vi "main.vi"() -> ()   [LabVIEW 2024]
uses:
  DataCluster.ctl
  <vilib>/userDefined/High Color/IMAQdx.ctl
  <vilib>/vision/Image Controls.llb/IMAQ Image.ctl
  <vilib>/Platform/TimedLoop/XDataNode/timing_clust.ctl
  <vilib>/Platform/TimedLoop/XDataNode/nitl_modes.ctl
  <vilib>/Platform/TimedLoop/XDataNode/wakeup.ctl
  4e5cdf46-f112-4ee0-b7be-49a859f3bfc5.vi
  <extravilib>/ChannelInstances/Tag-t'DataCluster.ctl'/Read With Abort.vi
  <extravilib>/ChannelInstances/Tag-t'DataCluster.ctl'/Write With Abort.vi
  <extravilib>/ChannelInstances/Tag-t'DataCluster.ctl'/Instantiate.vi
  <extravilib>/ChannelInstances/Tag-t'DataCluster.ctl'/EndpointRead.vi
  <extravilib>/ChannelInstances/Stream-str/Instantiate.vi
  <extravilib>/ChannelInstances/Tag-c(a[.](dbl),a[.](dbl))/Instantiate.vi
  <vilib>/Platform/browser.llb/Open URL in Default Browser (string).vi
  <extravilib>/ChannelInstances/Tag-t'DataCluster.ctl'/Endpoint.vi
  <vilib>/platform/TimedLoop/XDataNode/XDataNode.xnode
  <vilib>/vision/driver/NI_Vision_Acquisition_Software.lvlib
  <extravilib>/ChannelInstances/Tag-t'DataCluster.ctl'.lvlib
  <vilib>/Platform/TimedLoop/XDataNode/XDNodeRunTimeDep.lvlib
panel:
  out "Cooling label":string
  out "Galium Control":string="Galium Control" caption="Version"
  in  "Freeze":bool
  in  "Melt":bool
  in  "OverlayTemp?":bool
  out "error out 2":errorcluster
  out "T_Left":string="00:30:00" caption="Time Left:"
  out "version":string="version 0.0.0.1" caption="Version"
  in  "Start":bool
  out "Title":string="Ice Nucleation Contoller" caption="Version"
  out "Error Array":errorcluster[](array[cluster])
  out "cDAQ_Time":u32(graph) caption="DAQ - Process Time"
  out "DL_Time":u32(graph) caption="cDAQ - Process Time"
  out "DP_Overhead":i64(graph)=499 caption="Data Acquisition - Overhead"
  in  "DataCluster":T1={"Core"={"Current VI Reference"=refnum, "Close Panel on Exit?"=FALSE, "Exit"=FALSE, "Initialized?"=FALSE}, "Connections"={"cDAQ"={"Task"="", "Connected"=FALSE, "Active"=FALSE, "ID"=""}, "Camera"={"Session"="", "Connected"=FALSE, "Active"=FALSE, "Placeholder"=refnum}, "PSU"={"Port"="", "Connected"=FALSE, "Active"=FALSE}, "Arduino"={"Port"="", "Connected"=FALSE, "Active"=FALSE}}, "Data Acquisition"={"Setup"={"Label"="", "Operator"="", "Notes"="", "TempGrad"=0.0, "TargetTemp"=0.0, "Sample Volume"=1.0}, "Camera"={"Image"=refnum, "Save Image"=refnum, "Image Frequency"=20, "Rectangle"={"Left"=0, "Top"=0, "Right"=0, "Bottom"=0, "Rotation"=0.0}, "Calibration"={"Top Left"={"X"=0.0, "Y"=0.0}, "Top Right"={"X"=0.0, "Y"=0.0}, "Bottom Left"={"X"=0.0, "Y"=0.0}, "Bottom Right"={"X"=0.0, "Y"=0.0}, "Fixpoint"={"X"=0.0, "Y"=0.0}, "Scan Area"=0.0, "Fixpoint Area"=0.0, "Well Pixels"=[], "Valid"=FALSE}, "FocusPos"=0, "Display Mapping"=10, "Camera Mode"=10}, "Thermistor"={"Sample Size"=0, "Calibration"={"B0.100"=[], "R25"=[], "c"=[], "State"=[], "V_S"=0.0, "R_S"=0.0}, "Timing Mode"=14713}, "Partition"={"Data"=[], "Cell Label"="", "Cell Color"=0, "Height"=10, "Width"=16, "Grid"=[]}, "Queue"={"Size"=0, "Queue"=refnum}, "Sample Rate"=0, "Active"=FALSE, "Ready"=FALSE, "Graph Mode"=0, "Gradient Buffer"=2}, "Control"={"Sample Rate"=0, "PID gains"={"proportional gain (Kc)"=0.0, "integral time (Ti, min)"=0.0, "derivative time (Td, min)"=0.0}}, "Manual Temp Control"={"TargetTemp"=1.0, "Mode"=0, "Active"=FALSE}} {"Manual Temp Control"."Mode" items=["Cool", "Heat"]; "Manual Temp Control"."TargetTemp" min=-40.0 max=40.0 step=0.5 format="%#_g °C"; "Control"."PID gains"."derivative time (Td, min)" format="%.3f"; "Control"."PID gains"."integral time (Ti, min)" format="%.3f"; "Control"."PID gains"."proportional gain (Kc)" format="%.3f"; "Control"."Sample Rate" min=1 max=20 step=1 format="%.0f Samples/sec"; "Data Acquisition"."Gradient Buffer" min=2 max=30 step=1; "Data Acquisition"."Graph Mode" items=["Thermistor Temperature", "Camera Temperature"]; "Data Acquisition"."Thermistor"."Timing Mode" items=["Automatic"=16097, "High Resolution"=10195, "High Speed"=14712, "Best 50 Hz Rejection"=14713, "Best 60 Hz Rejection"=14714, "Custom"=10137]; "Data Acquisition"."Thermistor"."Calibration"."R_S" min=0.1 max=1000.0 format="%#_g kOhm"; "Data Acquisition"."Thermistor"."Calibration"."V_S" min=5.0 max=48.0 format="%#_g V"; "Data Acquisition"."Thermistor"."Calibration"."R25" min=0.1 max=1000.0 format="%#_g kOhm"; "Data Acquisition"."Thermistor"."Calibration"."B0.100" min=100.0 max=10000.0 format="%#_g K"; "Data Acquisition"."Thermistor"."Sample Size" min=1 max=200; "Data Acquisition"."Sample Rate" min=20 max=240 format="%.0f samples/min"; "Data Acquisition"."Queue"."Size" min=1 max=200; "Data Acquisition"."Camera"."Camera Mode" items=["Temperature Linear", "Signal Linear"]; "Data Acquisition"."Camera"."Display Mapping" items=["Default"=10, "Most Significant Bits"=11, "Full Dynamic"=12, "Downshift"=13, "Given Range"=14, "90% Dynamic"=15, "Given Percent Range"=16]; "Data Acquisition"."Camera"."Calibration"."Fixpoint"."Y" format="%.2f"; "Data Acquisition"."Camera"."Calibration"."Fixpoint"."X" format="%.2f"; "Data Acquisition"."Camera"."Calibration"."Top Left"."Y" format="%.2f"; "Data Acquisition"."Camera"."Calibration"."Top Left"."X" format="%.2f"; "Data Acquisition"."Camera"."Calibration"."Top Right"."Y" format="%.2f"; "Data Acquisition"."Camera"."Calibration"."Top Right"."X" format="%.2f"; "Data Acquisition"."Camera"."Calibration"."Bottom Left"."Y" format="%.2f"; "Data Acquisition"."Camera"."Calibration"."Bottom Left"."X" format="%.2f"; "Data Acquisition"."Camera"."Calibration"."Bottom Right"."Y" format="%.2f"; "Data Acquisition"."Camera"."Calibration"."Bottom Right"."X" format="%.2f"; "Data Acquisition"."Camera"."Rectangle"."Rotation" min=-90.0 max=90.0 step=1.0 format="%.2f"; "Data Acquisition"."Camera"."Rectangle"."Left" scale=0.0..1024.0; "Data Acquisition"."Camera"."Rectangle"."Right" scale=0.0..1024.0; "Data Acquisition"."Camera"."Image Frequency" min=1 max=60 step=1; "Data Acquisition"."Setup"."Sample Volume" min=0.0 max=500.0 format="%#_g µL"; "Data Acquisition"."Setup"."TargetTemp" min=-40.0 max=40.0 step=0.5 format="%#_g °C"; "Data Acquisition"."Setup"."TempGrad" min=-100.0 max=100.0 step=0.1 format="%#_g °C/min"}
  in  "Help":bool
  out "Temps":waveform(dbl)[](graph)=[{"t0"=timestamp(0 s since 1904-01-01), "dt"=0.5, "Y"=[0.0, 0.0, 0.0, 0.0, 0.0, 0.0, 0.0, 0.0, 0.0, 0.0, 0.0, 0.0, 0.0, 0.0, 0.0, 0.0, 0.0, 0.0, 0.0, 0.0, 0.0, 0.0, 0.0, 0.0, 0.0, 0.0, 0.0, 0.0, 0.0, 0.0, 0.0, 0.0, 0.0, 0.0, 0.0, 0.0, 0.0, 0.0, 0.0, 0.0, 0.0, 0.0, 0.0, 0.0, 0.0, 0.0, 0.0, 0.0, 0.0, 0.0, 0.0, 0.0, 0.0, 0.0, 0.0, 0.0, 0.0, 0.0, 0.0, 0.0, 0.0, 0.0, 0.0, 0.0, 0.0, 0.0, 0.0, 0.0, 0.0, 0.0, 0.0, 0.0, 0.0, 0.0, 0.0, 0.0, 0.0, 0.0, 0.0, 0.0, 0.0, 0.0, 0.0, 0.0, 0.0, 0.0, 0.0, 0.0, 0.0, 0.0, 0.0, 0.0, 0.0, 0.0, 0.0, 0.0, 0.0, 0.0, 0.0, 0.0, 0.0, 0.0, 0.0, 0.0, 0.0, 0.0, 0.0, 0.0, 0.0, 0.0, 0.0, 0.0, 0.0, 0.0, 0.0, 0.0, 0.0, 0.0, 0.0, 0.0, 0.0, 0.0, 0.0, 0.0, 0.0, 0.0, 0.0, 0.0, 0.0, 0.0, 0.0, 0.0, 0.0, 0.0, 0.0, 0.0, 0.0, 0.0, 0.0, 0.0, 0.0, 0.0, 0.0, 0.0]}, {"t0"=timestamp(0 s since 1904-01-01), "dt"=0.5, "Y"=[-30.0, -30.0, 40.0, 40.0, -30.0, 10.0, 10.0, -30.0, -30.0, -30.0, -30.0, -30.0, -30.0, -30.0, -30.0, -30.0, -30.0, -30.0, -30.0, -30.0, -30.0, -30.0, -30.0, -30.0, -30.0, -30.0, -30.0, -30.0, -30.0, -30.0, -30.0, -30.0, -30.0, -30.0, -30.0, -30.0, -30.0, -30.0, -30.0, -30.0, -30.0, -30.0, -30.0, -30.0, -30.0, -30.0, -30.0, -30.0, -30.0, -30.0, -30.0, -30.0, -30.0, -30.0, -30.0, -30.0, -30.0, -30.0, -30.0, -30.0, -30.0, -30.0, -30.0, -30.0, -30.0, -30.0, -30.0, -30.0, -30.0, -30.0, -30.0, -30.0, -30.0, -30.0, -30.0, -30.0, -30.0, -30.0, -30.0, -30.0, -30.0, -30.0, -30.0, -30.0, -30.0, -30.0, -30.0, -30.0, -30.0, -30.0, -30.0, -30.0, -30.0, -30.0, -30.0, -30.0, -30.0, -30.0, -30.0, -30.0, -30.0, -30.0, -30.0, -30.0, -30.0, -30.0, -30.0, -30.0, -30.0, -30.0, -30.0, 10.0, 10.0, 10.0, 10.0, 10.0, 10.0, -30.0, -30.0, -30.0, -30.0, -30.0, -30.0, -30.0, -30.0, -30.0, -30.0, -30.0, -30.0, -30.0, -30.0, -30.0, -30.0, -30.0, -30.0, -30.0, -30.0, -30.0, -30.0, -30.0, -30.0, -30.0, -30.0, -30.0]}]
  out "Gradients":waveform(dbl)[](graph)=[{"t0"=timestamp(0 s since 1904-01-01), "dt"=0.5, "Y"=[0.0, 0.0, 0.0, 0.0, 0.0, 0.0, 0.0, 0.0, 0.0, 0.0, 0.0, 0.0, 0.0, 0.0, 0.0, 0.0, 0.0, 0.0, 0.0, 0.0, 0.0, 0.0, 0.0, 0.0, 0.0, 0.0, 0.0, 0.0, 0.0, 0.0, 0.0, 0.0, 0.0, 0.0, 0.0, 0.0, 0.0, 0.0, 0.0, 0.0, 0.0, 0.0, 0.0, 0.0, 0.0, 0.0, 0.0, 0.0, 0.0, 0.0, 0.0, 0.0, 0.0, 0.0, 0.0, 0.0, 0.0, 0.0, 0.0, 0.0, 0.0, 0.0, 0.0, 0.0, 0.0, 0.0, 0.0, 0.0, 0.0, 0.0, 0.0, 0.0, 0.0, 0.0, 0.0, 0.0, 0.0, 0.0, 0.0, 0.0, 0.0, 0.0, 0.0, 0.0, 0.0, 0.0, 0.0, 0.0, 0.0, 0.0, 0.0, 0.0, 0.0, 0.0, 0.0, 0.0, 0.0, 0.0, 0.0, 0.0, 0.0, 0.0, 0.0, 0.0, 0.0, 0.0, 0.0, 0.0, 0.0, 0.0, 0.0, 0.0, 0.0, 0.0, 0.0, 0.0, 0.0, 0.0, 0.0, 0.0, 0.0, 0.0, 0.0, 0.0, 0.0, 0.0, 0.0, 0.0, 0.0, 0.0, 0.0, 0.0, 0.0, 0.0, 0.0, 0.0, 0.0, 0.0, 0.0, 0.0, 0.0, 0.0, 0.0, 0.0]}, {"t0"=timestamp(0 s since 1904-01-01), "dt"=0.5, "Y"=[-1.0, -1.0, -1.0, -1.0, -1.0, -1.0, -1.0, -1.0, -1.0, -1.0, -1.0, -1.0, -1.0, -1.0, -1.0, -1.0, -1.0, -1.0, -1.0, -1.0, -1.0, -1.0, -1.0, -1.0, -1.0, -1.0, -1.0, -1.0, -1.0, -1.0, -1.0, -1.0, -1.0, -1.0, -1.0, -1.0, -1.0, -1.0, -1.0, -1.0, -1.0, -1.0, -1.0, -1.0, -1.0, -1.0, -1.0, -1.0, -1.0, -1.0, -1.0, -1.0, -1.0, -1.0, -1.0, -1.0, -1.0, -1.0, -1.0, -1.0, -1.0, -1.0, -1.0, -1.0, -1.0, -1.0, -1.0, -1.0, -1.0, -1.0, -1.0, -1.0, -1.0, -1.0, -1.0, -1.0, -1.0, -1.0, -1.0, -1.0, -1.0, -1.0, -1.0, -1.0, -1.0, -1.0, -1.0, -1.0, -1.0, -1.0, -1.0, -1.0, -1.0, -1.0, -1.0, -1.0, -1.0, -1.0, -1.0, -1.0, -1.0, -1.0, -1.0, -1.0, -1.0, -1.0, -1.0, -1.0, -1.0, -1.0, -1.0, -1.0, -1.0, -1.0, -1.0, -1.0, -1.0, -1.0, -1.0, -1.0, -1.0, -1.0, -1.0, -1.0, -1.0, -1.0, -1.0, -1.0, -1.0, -1.0, -1.0, -1.0, -1.0, -1.0, -1.0, -1.0, -1.0, -1.0, -1.0, -1.0, -1.0, -1.0, -1.0, -1.0]}]
  out "Temp":dbl[unit] caption="Temperature" format="%.2f"
  out "Camera Feed":T3(plugin-control)
  out "Cooling%":dbl(slide) caption="Cooling" scale=0.0..100.0 scale format="%.0f %"
  out "StatusString":string="Closing System"
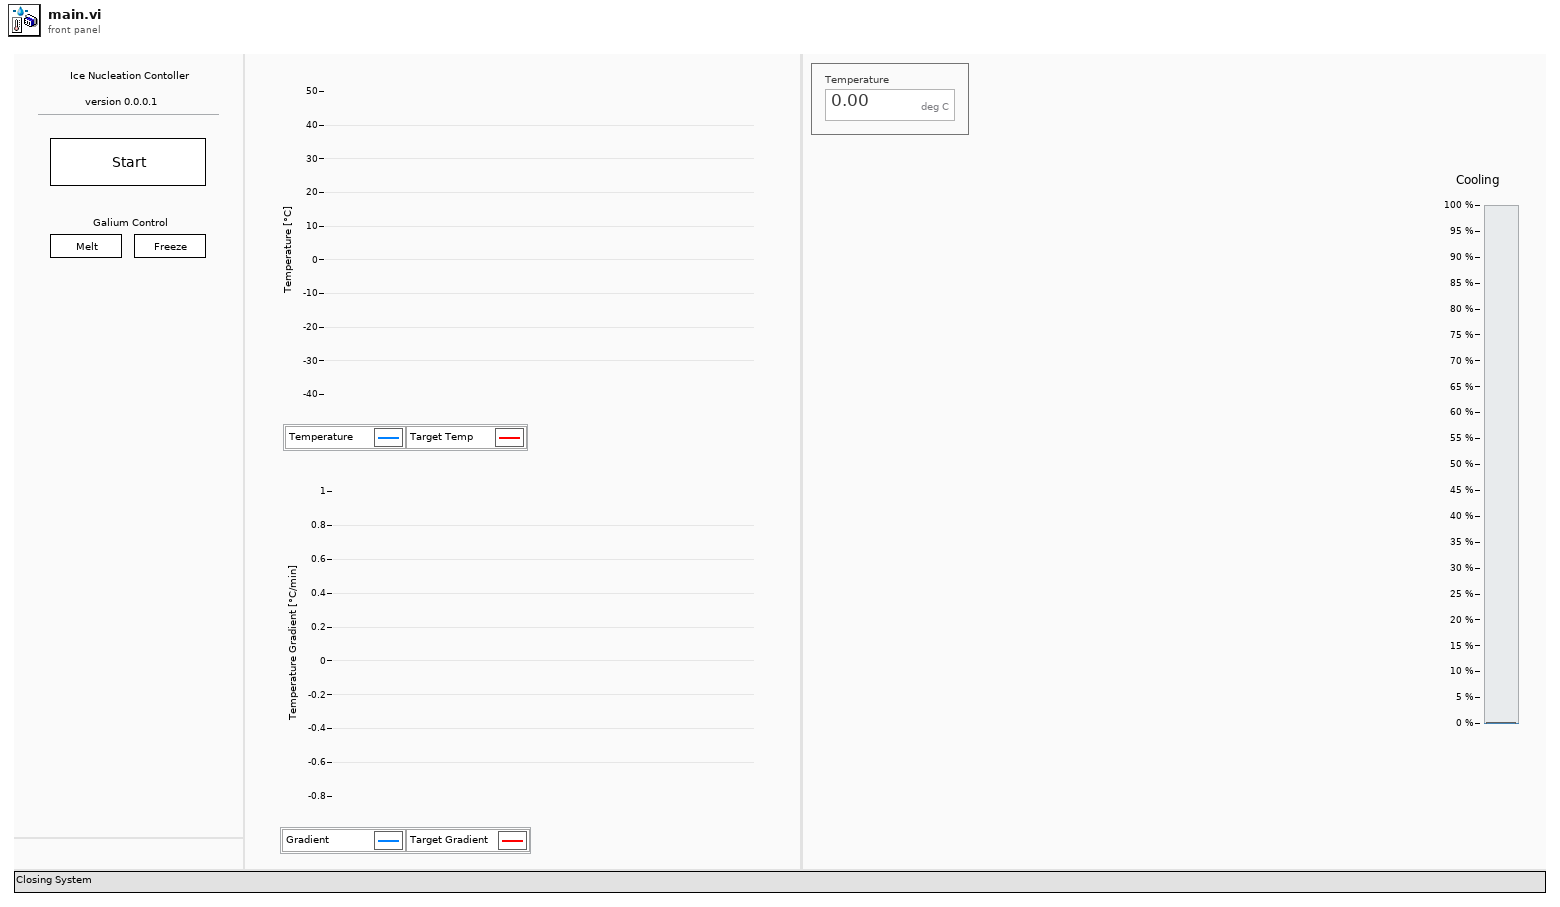
[diagram p1: front panel]
types:
  T1 = typedef "DataCluster.ctl" = cluster{"Core":cluster{"Current VI Reference":refnum<vi>, "Close Panel on Exit?":bool, "Exit":bool, "Initialized?":bool}, "Connections":cluster{"cDAQ":cluster{"Task":refnum<k21>, "Connected":bool, "Active":bool, "ID":string}, "Camera":cluster{"Session":T2, "Connected":bool, "Active":bool, "Placeholder":T3}, "PSU":cluster{"Port":refnum<visa-resource-name>, "Connected":bool, "Active":bool}, "Arduino":cluster{"Port":refnum<visa-resource-name>, "Connected":bool, "Active":bool}}, "Data Acquisition":cluster{"Setup":cluster{"Label":string, "Operator":string, "Notes":string, "TempGrad":dbl, "TargetTemp":dbl, "Sample Volume":dbl}, "Camera":cluster{"Image":T3, "Save Image":T3, "Image Frequency":i32, "Rectangle":T4, "Calibration":cluster{"Top Left":T5, "Top Right":T5, "Bottom Left":T5, "Bottom Right":T5, "Fixpoint":T5, "Scan Area":dbl, "Fixpoint Area":dbl, "Well Pixels":cluster{"X":i32, "Y":i32}[][], "Valid":bool}, "FocusPos":u32, "Display Mapping":u32, "Camera Mode":u32}, "Thermistor":cluster{"Sample Size":i32, "Calibration":cluster{"B0.100":dbl[], "R25":dbl[], "c":dbl[][], "State":bool[], "V_S":dbl, "R_S":dbl}, "Timing Mode":i32}, "Partition":cluster{"Data":string[][], "Cell Label":string, "Cell Color":u32, "Height":i32, "Width":i32, "Grid":string[][]}, "Queue":cluster{"Size":i32, "Queue":refnum<queue>}, "Sample Rate":i32, "Active":bool, "Ready":bool, "Graph Mode":u16, "Gradient Buffer":i32}, "Control":cluster{"Sample Rate":i32, "PID gains":cluster{"proportional gain (Kc)":dbl, "integral time (Ti, min)":dbl, "derivative time (Td, min)":dbl}}, "Manual Temp Control":cluster{"TargetTemp":dbl, "Mode":u16, "Active":bool}}
  T2 = typedef "IMAQdx.ctl" = refnum<k21>
  T3 = typedef "IMAQ Image.ctl" = refnum<image>
  T4 = typedef "IMAQ Rectangle" = cluster{"Left":i32, "Top":i32, "Right":i32, "Bottom":i32, "Rotation":dbl}
  T5 = typedef "IMAQ Point" = cluster{"X":sgl, "Y":sgl}
  T6 = enum32{"invalid app kind", "Development System", "Run Time System", "Student Edition", "Embedded LabVIEW", "Evaluation", "Custom"}
  T7 = enum32{"Invalid", "Standard", "Closed", "Hidden", "Minimized", "Maximized"}
  T8 = cluster{"Top Left":T5, "Top Right":T5, "Bottom Left":T5, "Bottom Right":T5, "Fixpoint":T5, "Scan Area":dbl, "Fixpoint Area":dbl, "Well Pixels":cluster{"X":i32, "Y":i32}[][], "Valid":bool}
  T9 = enum8{"Enabled", "Disabled", "Disabled and Grayed Out"}
  T10 = enum16{"Left Button", "Center Button", "Right Button", "Window Close"}
  T11 = cluster{"Current VI Reference":refnum<vi>, "Close Panel on Exit?":bool, "Exit":bool, "Initialized?":bool}
  T12 = cluster{"cDAQ":cluster{"Task":refnum<k21>, "Connected":bool, "Active":bool, "ID":string}, "Camera":cluster{"Session":T2, "Connected":bool, "Active":bool, "Placeholder":T3}, "PSU":cluster{"Port":refnum<visa-resource-name>, "Connected":bool, "Active":bool}, "Arduino":cluster{"Port":refnum<visa-resource-name>, "Connected":bool, "Active":bool}}
  T13 = typedef "Image Type" = u32
  T14 = typedef "Stream-str.lvlib/)Channel.ctl" = refnum<queue>
  T15 = typedef "Tag-t'DataCluster.ctl'.lvlib/))Channel.ctl" = refnum<queue>
  T16 = typedef "XDNodeRunTimeDep.lvlib/timing_clust.ctl" = cluster{"Expected End [f-1]":u64, "Actual End [f-1]":u64, "Finished Late? [f-1]":bool, "Expected End [i-1]":u64, "Actual End [i-1]":u64, "Finished Late? [i-1]":bool, "Expected Start [i]":u64, "Actual Start [i]":u64, "Expected Start [f]":u64, "Actual Start [f]":u64, "Source Name":string, "Structure Name":string, "Period":i64, "Deadline":i64, "Offset":i64, "Start":i64, "Priority":i32, "Timeout":i32, "Mode":T17, "Wakeup Reason":T18, "Error":errorcluster, "Source Type":string, "Secondary Source Type":string, "Global End Time":u64, "Global Start Time":u64, "Frame Duration":u64, "Iteration Duration":u64, "Assigned CPU":i32, "I/O Scan Engine Mode":u32}
  T17 = typedef "XDNodeRunTimeDep.lvlib/nitl_modes.ctl" = enum32{"No Change", "Process missed periods, maintain original phase", "Discard missed periods, maintain original phase", "Process missed periods, ignore original phase", "Discard missed periods, ignore original phase"}
  T18 = typedef "XDNodeRunTimeDep.lvlib/wakeup.ctl" = enum32{"Normal", "Aborted", "Asynchronous wakeup", "Timing source error", "Timed loop error", "Timeout"}
  T19 = typedef "Tag-c(a[.](dbl),a[.](dbl)).lvlib/))Channel.ctl" = refnum<queue>
  T20 = cluster{"Mean Temp":dbl[], "Target Temp":dbl[], "Temp Gradient":dbl[], "Target Gradient":dbl[], "Temperatures":dbl[][]}
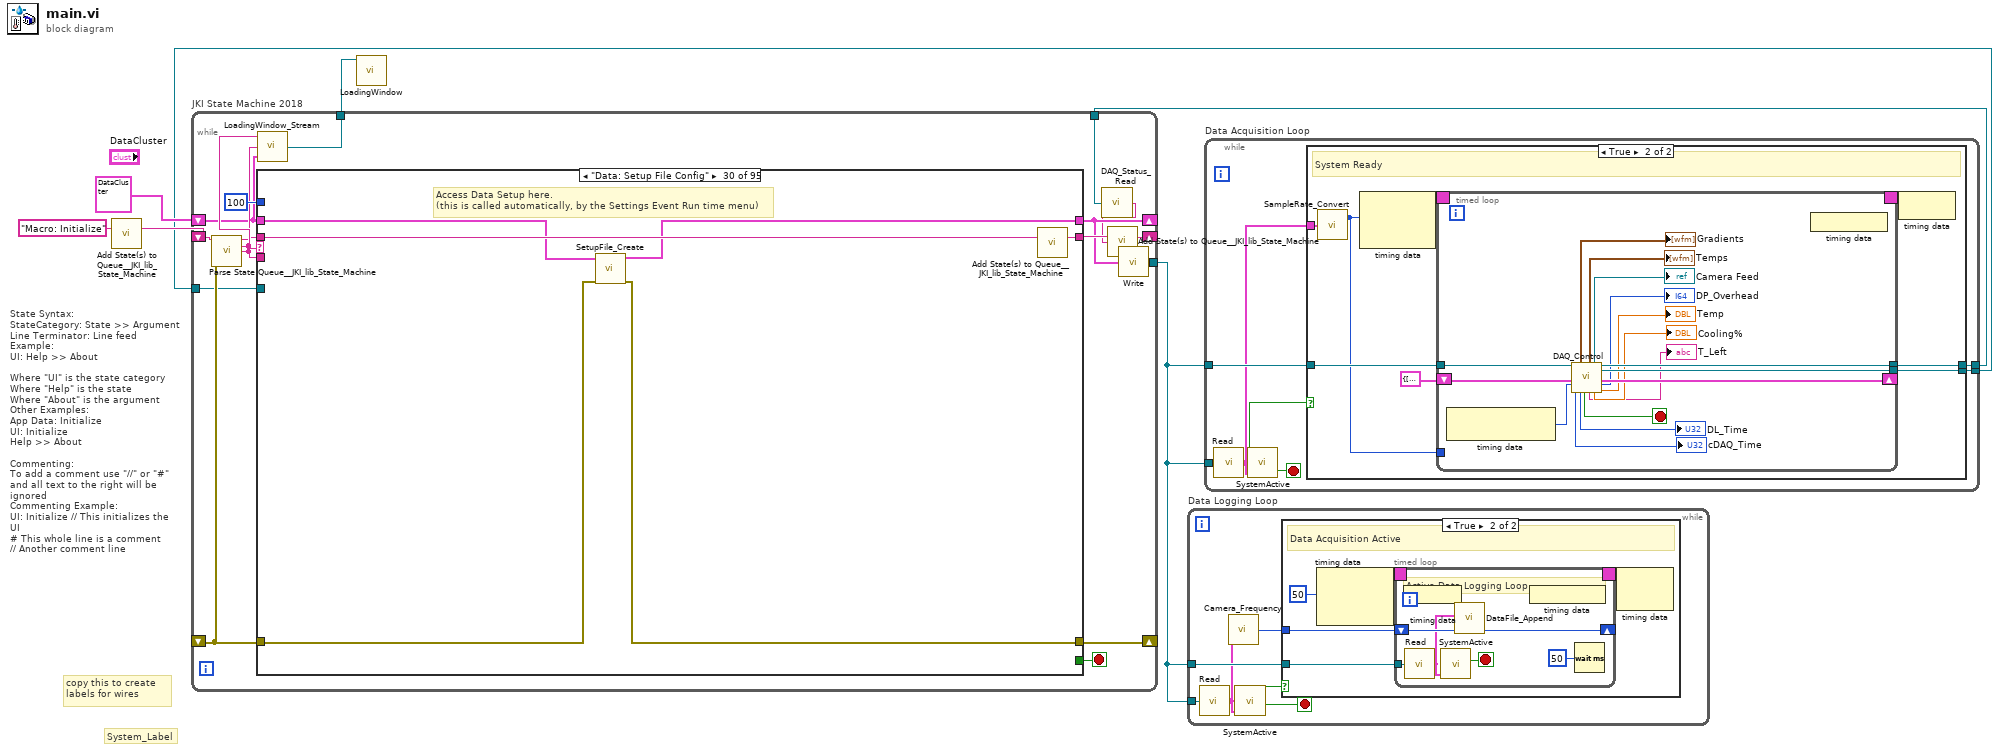
[diagram p0: block diagram]
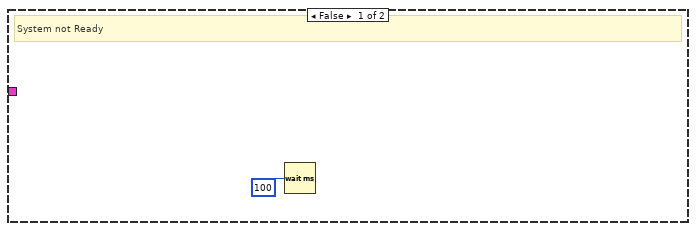
[diagram p2: hidden frame]
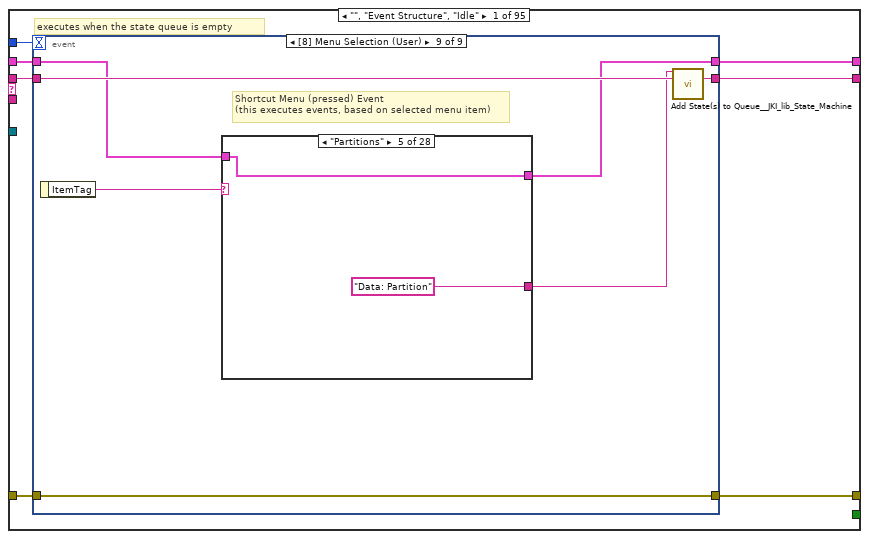
[diagram p3: hidden frame]
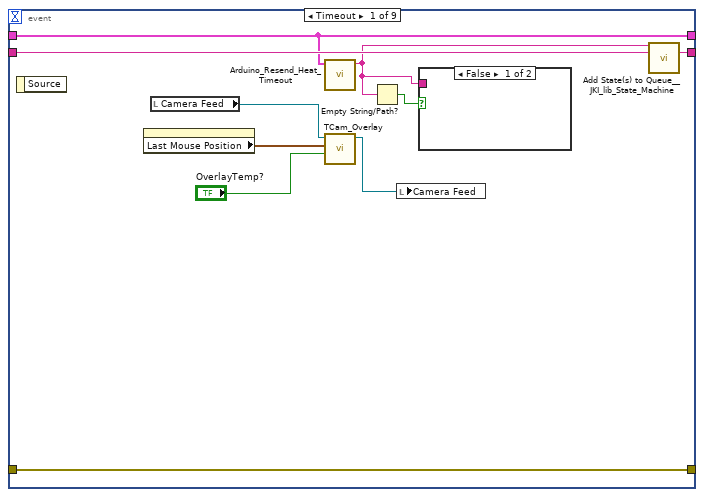
[diagram p4: hidden frame]
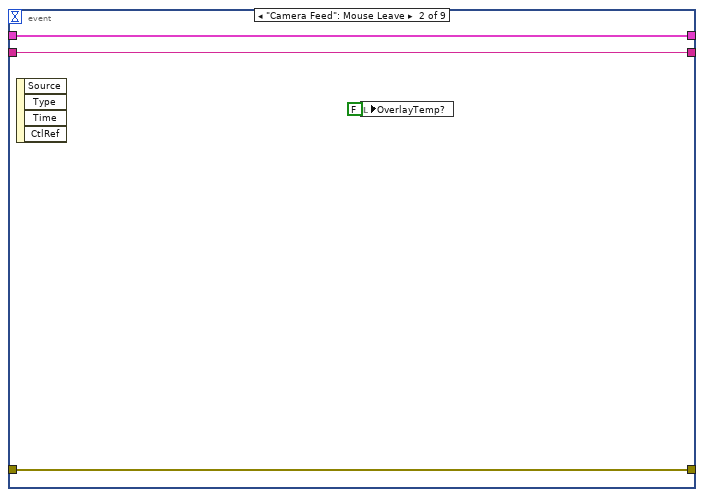
[diagram p6: hidden frame]
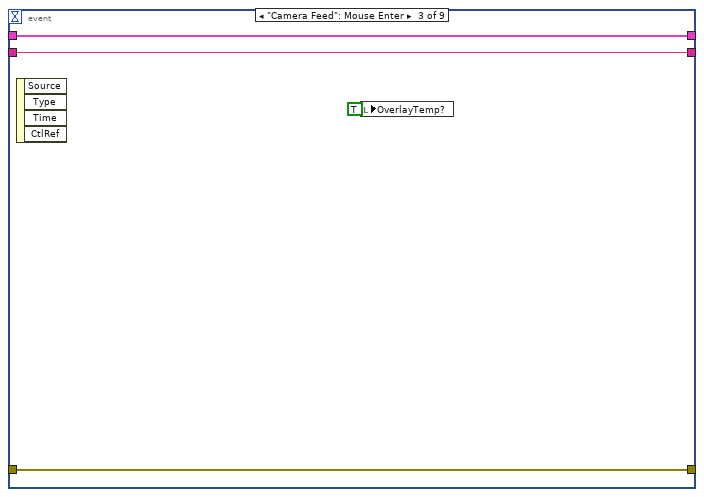
[diagram p7: hidden frame]
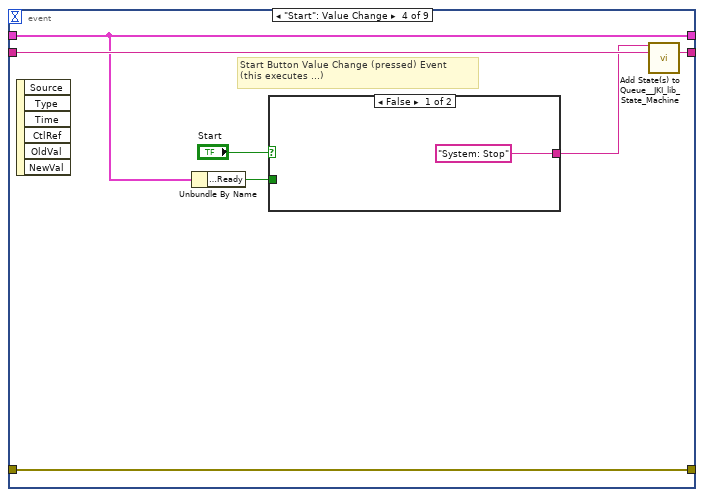
[diagram p8: hidden frame]
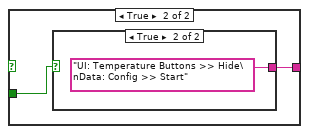
[diagram p9: hidden frame]
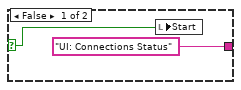
[diagram p10: hidden frame]
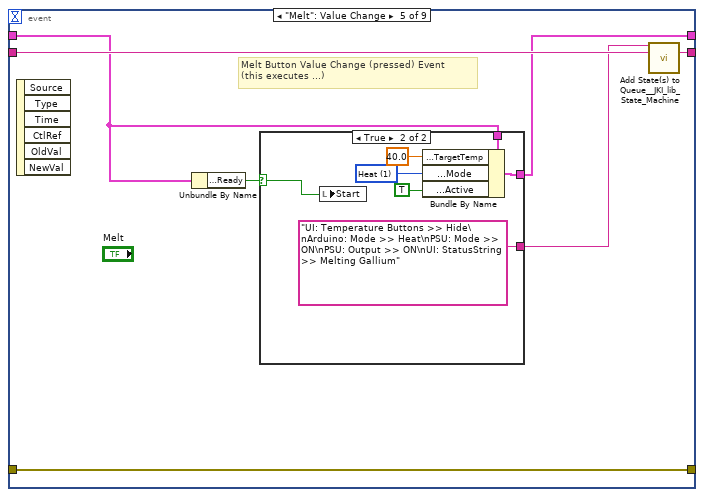
[diagram p11: hidden frame]
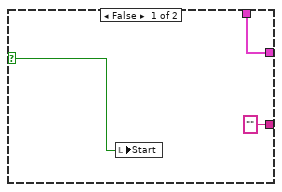
[diagram p12: hidden frame]
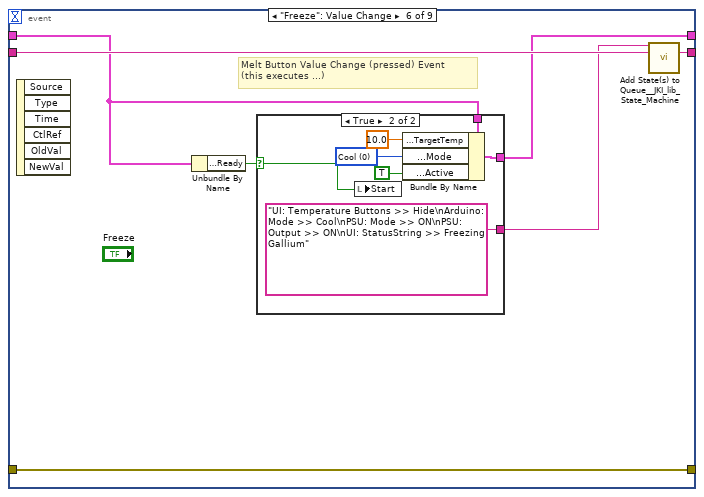
[diagram p13: hidden frame]
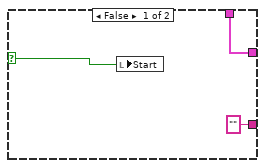
[diagram p14: hidden frame]
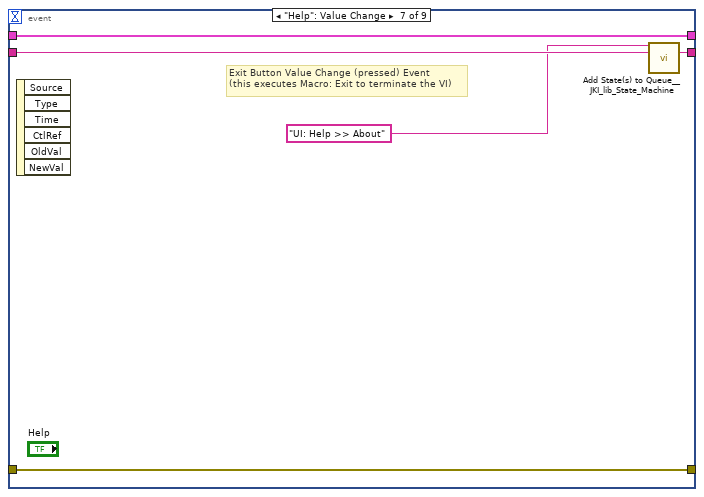
[diagram p15: hidden frame]
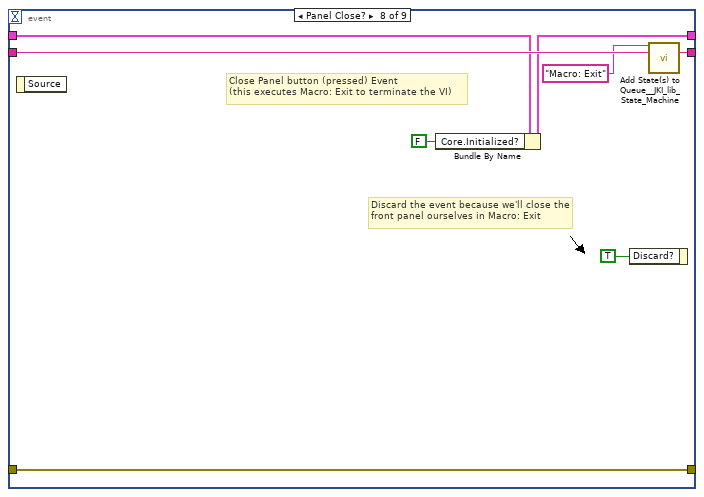
[diagram p16: hidden frame]
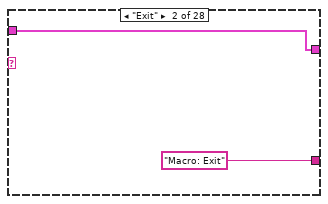
[diagram p18: hidden frame]
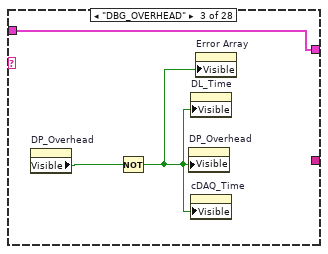
[diagram p19: hidden frame]
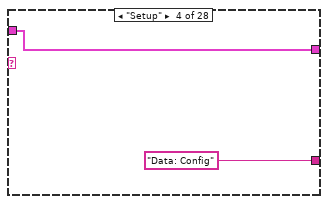
[diagram p20: hidden frame]
diagram:
  # "State Syntax:\nStateCategory: State >> Argument\nLine Terminator: Line feed\nExample:\nUI: Help >> About\n\nWhere \"UI\" is the state category\nWhere \"Help\" is the state\nWhere \"About\" is the argument\nOther Examples:\nApp Data: Initialize\nUI: Initialize\nHelp >> About\n\nCommenting:\nTo add a comment use \"//\" or \"#\" and all text to the right will be ignored\nCommenting Example:\nUI: Initialize // This initializes the UI\n# This whole line is a comment\n// Another comment line"
  # "copy this to create labels for wires"
  # "System_Label"
  n1 = call <vilib>:"Add State(s) to Queue__JKI_lib_State_Machine.vi"("State(s) in (\"\")"="Macro: Initialize") -> ("States Out"=w7:string)  [unwired: 14 in]
  n2 = while "JKI State Machine 2018" {
    shift-right: [w12] -> _
    shift-left: T1 {"Core"={"Current VI Reference"=refnum, "Close Panel on Exit?"=FALSE, "Exit"=FALSE, "Initialized?"=FALSE}, "Connections"={"cDAQ"={"Task"="", "Connected"=FALSE, "Active"=FALSE, "ID"=""}, "Camera"={"Session"="", "Connected"=FALSE, "Active"=FALSE, "Placeholder"=refnum}, "PSU"={"Port"="", "Connected"=FALSE, "Active"=FALSE}, "Arduino"={"Port"="", "Connected"=FALSE, "Active"=FALSE}}, "Data Acquisition"={"Setup"={"Label"="", "Operator"="", "Notes"="", "TempGrad"=0.0, "TargetTemp"=0.0, "Sample Volume"=1.0}, "Camera"={"Image"=refnum, "Save Image"=refnum, "Image Frequency"=20, "Rectangle"={"Left"=0, "Top"=0, "Right"=0, "Bottom"=0, "Rotation"=0.0}, "Calibration"={"Top Left"={"X"=0.0, "Y"=0.0}, "Top Right"={"X"=0.0, "Y"=0.0}, "Bottom Left"={"X"=0.0, "Y"=0.0}, "Bottom Right"={"X"=0.0, "Y"=0.0}, "Fixpoint"={"X"=0.0, "Y"=0.0}, "Scan Area"=0.0, "Fixpoint Area"=0.0, "Well Pixels"=[], "Valid"=FALSE}, "FocusPos"=0, "Display Mapping"=10, "Camera Mode"=10}, "Thermistor"={"Sample Size"=0, "Calibration"={"B0.100"=[], "R25"=[], "c"=[], "State"=[], "V_S"=0.0, "R_S"=0.0}, "Timing Mode"=14713}, "Partition"={"Data"=[], "Cell Label"="", "Cell Color"=0, "Height"=10, "Width"=16, "Grid"=[]}, "Queue"={"Size"=0, "Queue"=refnum}, "Sample Rate"=0, "Active"=FALSE, "Ready"=FALSE, "Graph Mode"=0, "Gradient Buffer"=2}, "Control"={"Sample Rate"=0, "PID gains"={"proportional gain (Kc)"=0.0, "integral time (Ti, min)"=0.0, "derivative time (Td, min)"=0.0}}, "Manual Temp Control"={"TargetTemp"=1.0, "Mode"=0, "Active"=FALSE}} ("DataCluster") -> [w9]
    shift-right: [w21] -> _
    shift-left: _ -> [w18]
    shift-right: [w15] -> _
    shift-left: w7 -> [w22]
    tunnel: [w17] -> w1
    tunnel: w4 -> [w14]
    tunnel: w3 -> [w13]
    tunnel: [w11] -> w2
    stop <- w20 stop-if-true
    n3 = call <vilib>:"Parse State Queue__JKI_lib_State_Machine.vi"("State Queue"=w22, "Error In (no error)"=w18) -> ("Remaining States"=w23:string, "Current State"=w24:string, "Arguments"=w10:string)  [unwired: 11 in]
    n4 = case shown="\"Data: Setup File Config\"" w24 {
      selector: w24 -> [_ _ w203 _ _ _ _ _ _ _ _ _ _ _ _ _ _ _ _ _ _ _ _ _ _ _ _ _ _ _ _ _ _ _ _ _ _ _ _ _ _ _ _ _ _ _ _ _ _ _ _ _ _ _ _ _ _ _ _ _ _ _ _ _ _ _ _ _ _ _ _ _ _ _ _ _ _ _ _ _ _ _ _ _ _ _ _ _ _ _ _ _ _ _ _]
      tunnel: w23 -> [w31 w202 w207 w223 w265 w274 w281 w285 w294 w307 w311 w320 w333 w342 w351 w364 w398 w411 w420 w433 w450 w458 w471 w482 w488 w495 w502 w505 w513 w519 w524 w548 w554 w568 w583 w591 w596 w605 w616 w628 w642 w647 w661 w666 w672 w679 w684 w693 w698 w709 w716 w733 w741 w771 w782 w851 w857 w861 w865 w869 w876 w880 w884 w889 w896 w904 w916 w922 w930 w942 w948 w955 w963 w975 w984 w1000 w1016 w1024 w1036 w1046 w1066 w1083 w1098 w1114 w1132 w1139 w1143 w1149 w1156 w1162 w1169 w1174 w1179 w1189 w1200]
      tunnel: w10 -> [_ _ _ w214 w255 _ _ _ _ _ _ _ w327 _ _ w358 _ _ _ _ _ w453 w466 _ _ _ _ _ _ _ _ _ _ _ _ _ _ _ _ _ _ w643 _ _ w668 _ w680 w689 w694 _ w712 w730 w737 w766 w776 _ _ _ _ _ _ _ _ _ _ _ _ _ _ _ _ w951 _ _ w982 w993 _ _ _ _ _ _ _ _ _ _ _ _ _ _ _ _ _ _ _]
      tunnel: w9 -> [w29 w199 w205 w219 w263 w271 w277 w282 w291 w296 w308 w312 w330 w338 w348 w357 w395 _ w417 w426 w438 w455 w468 w480 w485 w493 w500 w507 w509 w517 w522 w534 w550 w562 w572 w588 w593 w602 w610 w625 w636 w645 w659 w664 w669 w675 w682 w691 w696 w706 w714 w728 w739 w769 w778 w848 w854 w858 w862 w866 w873 w877 w881 w886 w893 w900 w913 w920 w926 w939 w946 w953 w959 w972 w978 w995 w1013 w1020 w1033 w1037 w1062 w1079 w1094 w1110 w1130 w1133 w1140 w1147 w1154 w1158 w1167 w1170 w1177 w1187 w1197]
      tunnel: [w28 w200 w209 w220 w258 errorcluster {"status"=FALSE, "code"=0, "source"=""} ("error out") w279 w283 w292 w305 w309 w318 w331 w340 w349 w362 w396 w403 w414 w430 w434 w456 w469 w477 w486 w490 w497 w503 w510 w515 w520 w532 w552 w555 w570 w589 w594 w603 w614 w626 w640 w644 w658 w663 w670 w677 w681 w690 w695 w707 w713 w731 w738 w767 w779 w849 w855 w859 w863 w867 w874 w878 w882 w887 w891 w898 w914 w917 w924 w940 w943 w949 w957 w973 w981 w998 w1011 w1018 w1034 w1039 w1063 w1080 w1095 w1106 w1128 w1135 w1141 w1145 w1152 w1159 w1165 w1171 w1175 w1186 w1198] -> w21
      tunnel: w18 -> [w27 w200 w208 w221 w258 w267 w279 w283 w292 w305 w309 w318 w331 w340 w349 w362 w396 w404 w416 w430 w436 w456 w469 w477 w486 w491 w498 w503 w511 w516 w521 w526 w551 w556 w571 w589 w594 w603 w614 w626 w640 w644 w658 w663 w670 w677 w681 w690 w695 w707 w713 w731 w738 w768 w780 w849 w855 w859 w863 w867 w874 w878 w882 w887 w890 w897 w914 _ w923 w940 _ _ w956 w973 w976 w992 w1010 w1017 w1034 w1039 w1056 w1077 w1092 w1111 w1129 w1136 w1141 w1146 w1153 w1160 w1166 w1172 w1176 w1186 w1198]
      tunnel: [w30 w201 w206 w222 w264 w273 w280 w284 w293 w306 w310 w319 w332 w341 w350 w363 w397 w410 w419 w432 w449 w457 w470 w481 w487 w494 w501 w508 w512 w518 w523 w547 w553 w567 w582 w590 w595 w604 w615 w627 w641 w646 w660 w665 w671 w678 w683 w692 w697 w708 w715 w732 w740 w770 w781 w850 w856 w860 w864 w868 w875 w879 w883 w888 w895 w903 w915 w921 w929 w941 w947 w954 w962 w974 w983 w999 w1015 w1023 w1035 w1045 w1065 w1082 w1097 w1113 w1131 w1138 w1142 w1148 w1155 w1161 w1168 w1173 w1178 w1188 w1199] -> w16
      tunnel: [_ _ _ _ _ _ TRUE _ _ _ _ _ _ _ _ _ _ _ _ _ _ _ _ _ _ _ _ _ _ _ _ _ _ _ _ _ _ _ _ _ _ _ _ _ _ _ _ _ _ _ _ _ _ _ _ _ _ _ _ _ _ _ _ _ _ _ _ _ _ _ _ _ _ _ _ _ _ _ _ _ _ _ _ _ _ _ _ _ _ _ _ _ _ _ _] -> w20
      tunnel: [w26 w199 w205 w219 w263 w271 w275 w282 w291 w295 w308 w312 w328 w338 w347 w360 w395 w409 w417 w431 w448 w454 w467 w479 w484 w492 w499 w506 w509 w514 w522 w534 w549 w562 w572 w588 w593 w598 w609 w625 w636 w645 w659 w664 w669 w675 w682 w691 w696 w706 w714 w728 w739 w769 w778 w848 w853 w858 w862 w866 w872 w877 w881 w885 w894 w899 w913 w919 w925 w939 w945 w952 w958 w972 w979 w995 w1014 w1019 w1033 w1041 w1061 w1078 w1096 w1109 w1127 w1133 w1140 w1147 w1151 w1157 w1164 w1170 w1177 w1187 w1197] -> w12
      tunnel: 100 ("Timeout") -> [w25 _ _ _ _ _ _ _ _ _ _ _ _ _ _ _ _ _ _ _ _ _ _ _ _ _ _ _ _ _ _ _ _ _ _ _ _ _ _ _ _ _ _ _ _ _ _ _ _ _ _ _ _ _ _ _ _ _ _ _ _ _ _ _ _ _ _ _ _ _ _ _ _ _ _ _ _ _ _ _ _ _ _ _ _ _ _ _ _ _ _ _ _ _ _]
      tunnel: w14 -> [_ _ _ _ _ _ _ _ _ _ _ _ _ _ _ _ _ _ _ _ _ _ _ _ _ _ _ _ _ _ _ _ _ _ _ _ _ _ _ _ _ _ _ _ _ _ _ _ _ _ _ _ _ _ _ _ _ _ _ _ _ _ _ _ _ _ _ _ _ _ _ _ _ _ _ _ _ _ _ _ _ _ _ _ _ _ _ w1144 _ _ _ _ _ _ _]
      frame "", "Event Structure", "Idle" {
        # "executes when the state queue is empty"
        n5 = event shown="[8] Menu Selection (User)" {
          selector: _ -> [_ _ _ _ _ _ _ _ _]
          dyn-events: _ -> [_ _ _ _ _ _ _ _ _]
          timeout: w25 -> [_ _ _ _ _ _ _ _ _]
          tunnel: w31 -> [w41 w42 w47 w56 w69 w86 w101 w109 w116]
          tunnel: [w40 w42 w47 w55 w68 w85 w100 w108 w115] -> w30
          tunnel: w29 -> [w35 w43 w48 w51 w65 w82 w98 w106 w111]
          tunnel: [w39 w44 w46 w54 w67 w84 w99 w107 w114] -> w28
          tunnel: w27 -> [w39 w44 w46 w54 w67 w84 w99 w107 w114]
          tunnel: [w35 w43 w48 w51 w64 w81 w98 w103 w110] -> w26
          event Timeout {
            n6 = event-data() -> ()  [unwired: 1 in, 1 out]
            n7 = property on="Camera Feed" class="ImageControl"() -> ("Last Mouse Position"=w38:cluster{"X":i32, "Y":i32})  [unwired: 2 in, 2 out]
            n8 = local read "Camera Feed"() -> (w37:T3)
            n9 = call "Arduino_Resend_Heat_Timeout.vi"("DataCluster"=w35) -> ("state out"=w33:string)  [unwired: 10 in]
            n10 = call "TCam_Overlay.vi"("OverlayTemp?"="OverlayTemp?", "Mouse pos"=w38, "img in"=w37) -> ("Image Out"=w36:T3)  [unwired: 7 in, 1 out]
            n11 = Empty String/Path?(string/path=w33) -> (empty?=w34:bool)
            n12 = local write "Camera Feed"(w36) -> ()
            n13 = case shown="False" w34 {
              tunnel: w33 -> [_ _]
              frame False {
              }
              frame True {
              }
            }
            n14 = call <vilib>:"Add State(s) to Queue__JKI_lib_State_Machine.vi"("State(s) in Front (\"\")"=w33, "State(s) in (\"\")"=w41) -> ("States Out"=w40:string)  [unwired: 13 in]
          }
          event "Camera Feed": Mouse Leave {
            n15 = event-data() -> ()  [unwired: 1 in, 4 out]
            n16 = local write "OverlayTemp?"(FALSE ("Display?")) -> ()
          }
          event "Camera Feed": Mouse Enter {
            n17 = event-data() -> ()  [unwired: 1 in, 4 out]
            n18 = local write "OverlayTemp?"(TRUE ("Display?")) -> ()
          }
          event "Start": Value Change {
            # "Start Button Value Change (pressed) Event\n(this executes ...)"
            n19 = event-data() -> ()  [unwired: 1 in, 6 out]
            n20 = Unbundle By Name(w51) -> ("Data Acquisition.Ready"=w50:bool)
            n21 = case shown="False" "Start" {
              tunnel: ["System: Stop" ("State(s) in Front (\"\")") w59] -> w52
              tunnel: w50 -> [_ w58]
              frame False {
              }
              frame True {
                n22 = case shown="True" w58 {
                  selector: w58 -> [w60 _]
                  tunnel: ["UI: Connections Status" ("State(s) in Front (\"\")") "UI: Temperature Buttons >> Hide\nData: Config >> Start" ("State(s) in Front (\"\")")] -> w59
                  frame False {
                    n23 = local write "Start"(w60) -> ()
                  }
                  frame True {
                  }
                }
              }
            }
            n24 = call <vilib>:"Add State(s) to Queue__JKI_lib_State_Machine.vi"("State(s) in Front (\"\")"=w52, "State(s) in (\"\")"=w56) -> ("States Out"=w55:string)  [unwired: 13 in]
          }
          event "Melt": Value Change {
            # "Melt Button Value Change (pressed) Event\n(this executes ...)"
            n25 = event-data() -> ()  [unwired: 1 in, 6 out]
            n26 = Unbundle By Name(w65) -> ("Data Acquisition.Ready"=w66:bool)
            n27 = case shown="True" w66 {
              selector: w66 -> [w70 w73]
              tunnel: w65 -> [w71 w79]
              tunnel: [w71 w78] -> w64
              tunnel: ["" "UI: Temperature Buttons >> Hide\nArduino: Mode >> Heat\nPSU: Mode >> ON\nPSU: Output >> ON\nUI: StatusString >> Melting Gallium"] -> w63
              frame False {
                n28 = local write "Start"(w70) -> ()
              }
              frame True {
                w76 = u16 1 items=["Cool", "Heat"] ("Mode")
                n29 = local write "Start"(w73) -> ()
                n30 = Bundle By Name(cluster=w79, "Manual Temp Control.TargetTemp"=40.0, "Manual Temp Control.Mode"=w76, "Manual Temp Control.Active"=TRUE) -> (w78:T1)
              }
            }
            n31 = call <vilib>:"Add State(s) to Queue__JKI_lib_State_Machine.vi"("State(s) in Front (\"\")"=w63, "State(s) in (\"\")"=w69) -> ("States Out"=w68:string)  [unwired: 13 in]
          }
          event "Freeze": Value Change {
            # "Melt Button Value Change (pressed) Event\n(this executes ...)"
            n32 = event-data() -> ()  [unwired: 1 in, 6 out]
            n33 = Unbundle By Name(w82) -> ("Data Acquisition.Ready"=w83:bool)
            n34 = case shown="True" w83 {
              selector: w83 -> [w87 w90]
              tunnel: w82 -> [w88 w96]
              tunnel: [w88 w95] -> w81
              tunnel: ["" "UI: Temperature Buttons >> Hide\nArduino: Mode >> Cool\nPSU: Mode >> ON\nPSU: Output >> ON\nUI: StatusString >> Freezing Gallium"] -> w80
              frame False {
                n35 = local write "Start"(w87) -> ()
              }
              frame True {
                w93 = u16 0 items=["Cool", "Heat"] ("Mode")
                n36 = local write "Start"(w90) -> ()
                n37 = Bundle By Name(cluster=w96, "Manual Temp Control.TargetTemp"=10.0, "Manual Temp Control.Mode"=w93, "Manual Temp Control.Active"=TRUE) -> (w95:T1)
              }
            }
            n38 = call <vilib>:"Add State(s) to Queue__JKI_lib_State_Machine.vi"("State(s) in Front (\"\")"=w80, "State(s) in (\"\")"=w86) -> ("States Out"=w85:string)  [unwired: 13 in]
          }
          event "Help": Value Change {
            # "Exit Button Value Change (pressed) Event\n(this executes Macro: Exit to terminate the VI)"
            n39 = event-data() -> ()  [unwired: 1 in, 6 out]
            n40 = call <vilib>:"Add State(s) to Queue__JKI_lib_State_Machine.vi"("State(s) in Front (\"\")"="UI: Help >> About" ("State(s) in Front (\"\")"), "State(s) in (\"\")"=w101) -> ("States Out"=w100:string)  [unwired: 13 in]
          }
          event Panel Close? {
            # "Discard the event because we'll close the front panel ourselves in Macro: Exit"
            # "Close Panel button (pressed) Event\n(this executes Macro: Exit to terminate the VI)"
            n41 = event-data() -> ()  [unwired: 1 in, 1 out]
            n42 = Bundle By Name(cluster=w106, "Core.Initialized?"=FALSE) -> (w103:T1)
            n43 = event-data("Discard?"=TRUE) -> ()  [unwired: 1 in, 1 out]
            n44 = call <vilib>:"Add State(s) to Queue__JKI_lib_State_Machine.vi"("State(s) in Front (\"\")"="Macro: Exit", "State(s) in (\"\")"=w109) -> ("States Out"=w108:string)  [unwired: 13 in]
          }
          event Menu Selection (User) {
            # "Shortcut Menu (pressed) Event\n(this executes events, based on selected menu item)"
            n45 = event-data() -> ("ItemTag"=w113:string)  [unwired: 1 in]
            n46 = case shown="\"Partitions\"" w113 {
              tunnel: [_ "Macro: Exit" _ "Data: Config" "Data: Partition" "Data: Open Folder" "Data: Options" "Data: Calibration" "Tools: Sensor Readout" "Tools: Manual Temp Control" "Tools: Calibrate Thermal Camera" "Tools: Focus Thermal Camera" "Tools: Camera Feed\nConnections: Status" w144 w146 "UI: Chart Clear\nUI: Chart Setup" "UI: Cursor Set >> Busy\nConnections: Terminate\nConnections: Initialize\nUI: Cursor Set >> Idle" "System: Override" "UI: Connections Status" "UI: Cursor Set >> Busy\nUI: StatusString >> Checking for Updates\nCore: Check Update >> Display\nUI: StatusString >> Idle\nUI: Cursor Set >> Idle" _ _ _ _ "UI: Help >> About" "System: State >> OFF\nTools: PID\nSystem: State >> ON\nUI: Chart Setup\nUI: Chart Clear" w171 w185] -> w112
              tunnel: w111 -> [w117 w118 w122 w123 w125 w127 w129 w131 w133 w135 w137 w139 w141 w143 w145 w147 w149 w151 w153 w155 w157 w160 w163 w166 w167 w169 w173 w187]
              tunnel: [w117 w118 w122 w123 w125 w127 w129 w131 w133 w135 w137 w139 w141 w143 w145 w147 w149 w151 w153 w155 w157 w159 w162 w165 w167 w169 w172 w186] -> w110
              frame "False", Default {
              }
              frame "Exit" {
              }
              frame "DBG_OVERHEAD" {
                n47 = property on="DP_Overhead" class="WFChart (strict)"() -> ("Visible"=w121:bool)  [unwired: 2 in, 2 out]
                n48 = Not(x=w121) -> (.not. x?=w120:bool)
                n49 = property on="DP_Overhead" class="WFChart (strict)"("Visible"=w120) -> ()  [unwired: 2 in, 2 out]
                n50 = property on="DL_Time" class="WFChart (strict)"("Visible"=w120) -> ()  [unwired: 2 in, 2 out]
                n51 = property on="cDAQ_Time" class="WFChart (strict)"("Visible"=w120) -> ()  [unwired: 2 in, 2 out]
                n52 = property on="Error Array" class="Arr (strict)"("Visible"=w120) -> ()  [unwired: 2 in, 2 out]
              }
              frame "Setup" {
              }
              frame "Partitions" {
              }
              frame "Open Folder" {
              }
              frame "Options" {
              }
              frame "Calibration" {
              }
              frame "Manual Reading" {
              }
              frame "Temperature Control" {
              }
              frame "Thermal Cam Calibration" {
              }
              frame "Thermal Cam Focus" {
              }
              frame "Camera Feed" {
              }
              frame "Freeze Check" {
                w144 = "Tools: Freeze Check"  # Tools: Freeze Check
              }
              frame "Tool_TempCalc" {
                w146 = "Tools: Temp Calc"  # Tools: Temp Calc
              }
              frame "Reset Graph" {
              }
              frame "Reconnect" {
              }
              frame "System Override" {
              }
              frame "Status" {
              }
              frame "HELP_UPDATE" {
              }
              frame "HELP_MANUAL" {
                n53 = call-poly <vilib>:"Open URL in Default Browser.vi"("URL"="https://github.com/Aarhus-University-MPE/Ice-Nucleation-Controller/raw/main/docs/manual.pdf") -> ()  [unwired: 5 in, 2 out]
              }
              frame "TCAM_NUC" {
                n54 = call "TCam_NUC.vi"("DataCluster in"=w160) -> ("DataCluster out"=w159:T1)  [unwired: 9 in, 1 out]
              }
              frame "TCAM_NUC_ENABLE" {
                n55 = call "TCam_NUC_SET.vi"("Enable"=TRUE, "DataCluster in"=w163) -> ("DataCluster out"=w162:T1)  [unwired: 8 in, 1 out]
              }
              frame "TCAM_NUC_DISABLE" {
                n56 = call "TCam_NUC_SET.vi"("Enable"=FALSE, "DataCluster in"=w166) -> ("DataCluster out"=w165:T1)  [unwired: 8 in, 1 out]
              }
              frame "HELP_ABOUT" {
              }
              frame "PID_TUNE" {
              }
              frame "TEMP_MELT" {
                n57 = Unbundle By Name(w173) -> ("Data Acquisition.Ready"=w174:bool)
                n58 = case shown="True" w174 {
                  selector: w174 -> [w175 w178]
                  tunnel: w173 -> [w176 w184]
                  tunnel: [w176 w183] -> w172
                  tunnel: ["" "Arduino: Mode >> Heat\nPSU: Mode >> ON\nPSU: Output >> ON\nUI: StatusString >> Melting Gallium"] -> w171
                  frame False {
                    n59 = local write "Start"(w175) -> ()
                  }
                  frame True {
                    w181 = u16 1 items=["Cool", "Heat"] ("Mode")
                    n60 = local write "Start"(w178) -> ()
                    n61 = Bundle By Name(cluster=w184, "Manual Temp Control.TargetTemp"=40.0, "Manual Temp Control.Mode"=w181, "Manual Temp Control.Active"=TRUE) -> (w183:T1)
                  }
                }
              }
              frame "TEMP_FREEZE" {
                n62 = Unbundle By Name(w187) -> ("Data Acquisition.Ready"=w188:bool)
                n63 = case shown="True" w188 {
                  selector: w188 -> [w189 w192]
                  tunnel: w187 -> [w190 w198]
                  tunnel: [w190 w197] -> w186
                  tunnel: ["" "Arduino: Mode >> Cool\nPSU: Mode >> ON\nPSU: Output >> ON\nUI: StatusString >> Freezing Gallium"] -> w185
                  frame False {
                    n64 = local write "Start"(w189) -> ()
                  }
                  frame True {
                    w195 = u16 0 items=["Cool", "Heat"] ("Mode")
                    n65 = local write "Start"(w192) -> ()
                    n66 = Bundle By Name(cluster=w198, "Manual Temp Control.TargetTemp"=10.0, "Manual Temp Control.Mode"=w195, "Manual Temp Control.Active"=TRUE) -> (w197:T1)
                  }
                }
              }
            }
            n67 = call <vilib>:"Add State(s) to Queue__JKI_lib_State_Machine.vi"("State(s) in Front (\"\")"=w112, "State(s) in (\"\")"=w116) -> ("States Out"=w115:string)  [unwired: 13 in]
          }
        }
      }
      frame "---------- Core ----------" {
        # "Do not put any code in this frame.\n(it is a separator no-op)"
        n68 = call <vilib>:"Add State(s) to Queue__JKI_lib_State_Machine.vi"("State(s) in (\"\")"=w202) -> ("States Out"=w201:string)  [unwired: 14 in]
      }
      frame Default {
        w212 = 42 items=["No error", "Argument error", "Memory is full", "Out of zone", "End of file", "File already open", "Generic file I/O error", "File not found", "File permission error", "Disk is full", "Duplicate path", "Too many files open", "System feature not enabled", "Resource file not found", "Cannot add resource", "Resource not found", "Image not found", "Image memory error", "Pen does not exist", "Config type invalid", "Config token not found", "Config parse error", "Config memory error", "Bad external code format", "Bad external code offset", "External code not present", "Null window", "Destroy window error", "Null menu", "Print aborted", "Bad print record", "Print driver error", "Windows error during printing", "Memory error during printing", "Print dialog error", "Generic print error", "Invalid device refnum", "Device not found", "Device parameter error", "Device unit error", "Cannot open device", "Device call aborted", "Generic error", "Cancelled by user", "Object ID too low", "Object ID too high", "Object not in heap", "Unknown heap", "Unknown object (invalid DefProc)", "Unknown object (DefProc not in table)", "Message out of range", "Invalid (null) method", "Unknown message", "Manager call not supported", "Bad address", "Network operation in progress", "Network operation timed out", "Connection is busy", "Network attribute not supported", "Network error", "Address in use", "System out of memory", "Connection aborted", "Connection refused", "Not connected", "Already connected", "Connection closed", "Initialization error (interapplication manager)", "Bad occurrence", "Wait on unbound occurrence handler", "Occurrence queue overflow", "Datalog type conflict", "Unused", "Unrecognized type (interapplication manager)", "Memory corrupt", "Failed to make temporary DLL", "Old CIN version", "Drag socket not found", "Failed to load drop-object", "Failed to register OLE object", "Failed to release OLE object", "Format specifier type mismatch", "Unknown format specifier", "Too few format specifiers", "Too many format specifiers", "Scan failed", "Newer CIN version", "Error converting to variant", "Runtime menu error", "Password tampered", "Variant attribute not found", "Incompatible variant data type", "Event data is not available", "Event Store is not present", "Occurrence is not found", "Event Queue is not created", "Event info is not available", "Refnum passed is NULL", "Error retrieving Class GUID", "Error retrieving CoClass GUID", "Error retrieving TypeLib GUID.", "Bad built application magic bytes.", "Specific driver is different from the specific driver associated with the Logical Name.", "There is no session opened to the class driver.", "Max Error", "MAX - Error with config objects", "MAX - Error loading configuration", "MAX - Group not supported"]
        # "Current State"
        # "Do not delete, rename, or modify this frame.\n(this is used to capture unhandled states and typos)"
        # "Handle mistyped state name (developer tool)"
        n69 = Format Into String(format string="Software Exception: Unhandled State \"%s\"." ("message"), error in=w208, w203) -> (resulting string=w211:string, error out=w210:errorcluster)  [unwired: 1 in]
        n70 = call <vilib>:"Error Cluster From Error Code.vi"("show call chain? (False)"=TRUE, "error in (no error)"=w210, "error message (\"\")"=w211, "error code (0)"=w212) -> ("error out"=w209:errorcluster)  [unwired: 5 in]
        n71 = call <vilib>:"Add State(s) to Queue__JKI_lib_State_Machine.vi"("State(s) in (\"\")"=w207) -> ("States Out"=w206:string)  [unwired: 14 in]
      }
      frame "Core: Check Update" {
        # "exe?"
        # "Do not delete, rename, or modify this frame.\n(this is used to capture unhandled states and typos)"
        n72 = property class="App"() -> ("App.Kind"=w217:T6)  [unwired: 2 in, 2 out]
        n73 = Equal?(x=w217, y=T6."Run Time System" ("Application:Kind")) -> (x = y?=w216:bool)
        n74 = case shown="True" w216 {
          tunnel: w221 -> [w225 w235]
          tunnel: [w225 w234] -> w220
          tunnel: ["Loading UI: Version >> Version - x.x.x.x (32 bit) - Built on MM DD YYYY" w230] -> w215
          tunnel: w214 -> [_ w229]
          frame False {
          }
          frame True {
            n75 = call "Read Exe Version.vi"("Application name"=path "INC.exe") -> ("Build Date"=w236:string, "FileVersion"=w227:string)  [unwired: 7 in, 2 out]
            n76 = call "VersionCheck.vi"("error in (no error)"=w235, "Version"=w227) -> ("error out"=w234:errorcluster, "outdated?"=w226:bool, "Latest Version"=w228:string)  [unwired: 3 in]
            n77 = case shown="\"Display\"" w229 {
              tunnel: w227 -> [_ w242]
              tunnel: w226 -> [_ w241]
              frame "False", Default {
              }
              frame "Display" {
                # "Display up to date prompt?"
                n78 = case shown="False" w241 {
                  tunnel: w242 -> [w243 _]
                  frame False {
                    n79 = Concatenate Strings("Current version is the latest (" ("message"), w243, ")" ("string")) -> (w244:string)
                    n80 = One Button Dialog(message=w244) -> ()  [unwired: 1 in, 1 out]
                  }
                  frame True {
                  }
                }
              }
            }
            n81 = Concatenate Strings("version " ("string"), w227) -> (→"version":string)
            n82 = case shown="False" w226 {
              tunnel: ["" w248] -> w231
              tunnel: w228 -> [_ w249]
              frame False {
              }
              frame True {
                n83 = Concatenate Strings("\nCore: Update >> " ("string"), w249) -> (w248:string)
              }
            }
            n84 = Concatenate Strings("Loading UI: Version >> Version - " ("string"), w227, " (32 bit) - Built on " ("string"), w236) -> (w232:string)
            n85 = call <vilib>:"Add State(s) to Queue__JKI_lib_State_Machine.vi"("State(s) in Front (\"\")"=w232, "State(s) in (\"\")"=w231) -> ("States Out"=w230:string)  [unwired: 13 in]
          }
        }
        n86 = call <vilib>:"Add State(s) to Queue__JKI_lib_State_Machine.vi"("State(s) in Front (\"\")"=w215, "State(s) in (\"\")"=w223) -> ("States Out"=w222:string)  [unwired: 13 in]
      }
      frame "Core: Update" {
        # "Do not delete, rename, or modify this frame.\n(this is used to capture unhandled states and typos)"
        n87 = call "Read Exe Version.vi"("Application name"=path "INC.exe") -> ("FileVersion"=w253:string)  [unwired: 7 in, 3 out]
        n88 = Concatenate Strings("Current version: " ("message"), w253, "\nLateset version: " ("string"), w255, "\nUpdate to newest version?" ("string")) -> (w257:string)
        n89 = call <vilib>:"Three Button Dialog.vi"("Allow user to close window? (TRUE)"=FALSE, "Window Title (\"\")"="Update?" ("Window Title (\"\")"), "Right Button Text (\"Cancel\")"="Ignore update" ("Right Button Text (\"Cancel\")"), "message"=w257) -> ("Which Button?"=w252:T10)  [unwired: 7 in]
        n90 = case shown="\"Left Button\", Default" w252 {
          frame "Left Button", Default {
            n91 = call-poly <vilib>:"Open URL in Default Browser.vi"("URL"="https://github.com/MadsR/Ice-Nucleation/releases/latest") -> ()  [unwired: 5 in, 2 out]
          }
          frame "Center Button" {
          }
        }
        n92 = call <vilib>:"Add State(s) to Queue__JKI_lib_State_Machine.vi"("State(s) in (\"\")"=w265) -> ("States Out"=w264:string)  [unwired: 14 in]
      }
      frame "Error Handler" {
        # "Handle any errors here.\nYou can also output any states to clean-up after errors occur"
        # "Clear error"
        n93 = local read "Error Array"() -> (w268:errorcluster[])
        n94 = Build Array (concatenate)(w267, w268) -> (→"Error Array":errorcluster[])
        n95 = call <vilib>:"Add State(s) to Queue__JKI_lib_State_Machine.vi"("State(s) in Front (\"\")"="/* Post Error States", "State(s) in (\"\")"=w274) -> ("States Out"=w273:string)  [unwired: 13 in]
      }
      frame "Exit" {
        # "Do not put any code in this frame.\n(No errors that occur here will be handled.)"
        n96 = Bundle By Name(cluster=w277, "Core.Exit"=TRUE) -> (w275:T1)
        n97 = call <vilib>:"Add State(s) to Queue__JKI_lib_State_Machine.vi"("State(s) in (\"\")"=w281) -> ("States Out"=w280:string)  [unwired: 14 in]
      }
      frame "---------- Macro ----------" {
        # "Do not put any code in this frame.\n(It is a separator no-op. You can make a copy of this frame to create a new Macro frame)"
        n98 = call <vilib>:"Add State(s) to Queue__JKI_lib_State_Machine.vi"("State(s) in (\"\")"=w285) -> ("States Out"=w284:string)  [unwired: 14 in]
      }
      frame "Macro: Initialize" {
        # "Initialization Macro\n(This is called once, when the VI starts)"
        n99 = Current VI's Path() -> (path=w288:path)
        n100 = Open VI Reference(vi path=w288) -> (vi reference=w289:refnum<vi>)  [unwired: 5 in, 1 out]
        n101 = invoke class="VI" method="FP.Open"(reference=w289, "State"=T7."Hidden") -> (reference out=w286:refnum<vi>)  [unwired: 3 in, 4 out]
        n102 = Close Reference(reference=w286) -> ()  [unwired: 1 in, 1 out]
        n103 = call <vilib>:"Add State(s) to Queue__JKI_lib_State_Machine.vi"("State(s) in Front (\"\")"="UI: StatusString >> Initializing...\nUI: Cursor Set >> Busy\nUI: Start Button >> Connecting\nUI: StatusString >> Initializing Data\nData: Initialize\nLoading UI: Progress\nUI: StatusString >> Initializing Core Data\nData: Initialize Core Data\nLoading UI: Progress\nUI: StatusString >> Checking for Updates\nCore: Check Update\nLoading UI: Progress\nUI: StatusString >> Loading Thermistor Calibration\nData: Load Calibration\nLoading UI: Progress\nUI: StatusString >> Loading Camera Calibration\nData: Load Thermal Calibration\nUI: StatusString >> Initializing User Interface\nUI: Initialize\nLoading UI: Progress\nUI: StatusString >> Initializing Connections\nConnections: Initialize\nLoading UI: Progress\nUI: StatusString >> Finishing Initialization\nLoading UI: Exit\nUI: Front Panel State >> Maximized\nUI: Cursor Set >> Idle\nUI: StatusString >> Idle", "State(s) in (\"\")"=w294) -> ("States Out"=w293:string)  [unwired: 13 in]
      }
      frame "Macro: Exit" {
        # "Exit Macro\n(This is called once, when the VI exits)"
        n104 = Unbundle By Name(w296) -> ("Core.Close Panel on Exit?"=w304:bool)
        n105 = Bundle By Name(cluster=w296, "Data Acquisition.Ready"=FALSE) -> (w295:T1)
        n106 = Select(t="UI: Front Panel State >> Close", s=w304, f="") -> (s? t:f=w301:string)
        n107 = call <vilib>:"Add State(s) to Queue__JKI_lib_State_Machine.vi"("State(s) in Front (\"\")"="UI: StatusString >> Closing System... Terminating Data Acquisition\nSystem: Stop\nUI: StatusString >> Closing System... Terminating Connections\nConnections: Terminate\nUI: StatusString >> Closing System... Data Cleanup\nData: Terminate\nUI: StatusString >> Closing System" ("State(s) in Front (\"\")"), "State(s) in (\"\")"=w301, "State(s) at Back (\"\")"="Exit") -> ("States Out"=w300:string)  [unwired: 12 in]
        n108 = call <vilib>:"Add State(s) to Queue__JKI_lib_State_Machine.vi"("State(s) in Front (\"\")"=w300, "State(s) in (\"\")"=w307) -> ("States Out"=w306:string)  [unwired: 13 in]
      }
      frame "---------- System ----------" {
        # "Template Separator\n(You can make a copy of, or modify, this frame)"
        n109 = call <vilib>:"Add State(s) to Queue__JKI_lib_State_Machine.vi"("State(s) in (\"\")"=w311) -> ("States Out"=w310:string)  [unwired: 14 in]
      }
      frame "System: Start" {
        # "Your code here.\n(You can make a copy of, or modify, this frame)"
        n110 = Unbundle By Name(w312) -> ("Data Acquisition.Ready"=w314:bool, "Data Acquisition.Active"=w315:bool)
        n111 = Not(x=w315) -> (.not. x?=w313:bool)
        n112 = And(x=w314, y=w313) -> (x .and. y?=w316:bool)
        n113 = case shown="True" w316 {
          selector: w316 -> [w323 _]
          tunnel: [w322 "UI: Cursor Set >> Busy \nUI: StatusString >> Clearing Chart\nUI: Chart Setup\nUI: Chart Clear\n// ----------- Data Files Setup ----------- //\nUI: StatusString >> Configuring Setup file\nData: Setup File Config\nUI: StatusString >> Configuring Data file\nData: Data File Config\nUI: StatusString >> Configuring Image Folder\nData: Image Folder Setup\n// ----------- Data Acquisition Setup----------- //\nUI: StatusString >> Initializing Buffer\nData Acquisition: Buffer Initialize\nUI: StatusString >> Initializing Power Systems\nSystem: Power Initialize\nData Acquisition: Start\nUI: StatusString >> System Active\nUI: Time Left >> show\nUI: Cursor Set >> Idle" ("State(s) in Front (\"\")")] -> w317
          tunnel: w314 -> [w321 _]
          frame False {
            n114 = local write "Start"(w323) -> ()
            n115 = case shown="False" w321 {
              tunnel: ["UI: Connections Status" ("State(s) in Front (\"\")") "" ("State(s) in Front (\"\")")] -> w322
              frame False {
              }
              frame True {
              }
            }
          }
          frame True {
          }
        }
        n116 = call <vilib>:"Add State(s) to Queue__JKI_lib_State_Machine.vi"("State(s) in Front (\"\")"=w317, "State(s) in (\"\")"=w320) -> ("States Out"=w319:string)  [unwired: 13 in]
      }
      frame "System: State" {
        # "Your code here.\n(You can make a copy of, or modify, this frame)"
        n117 = case shown="\"OFF\"" w327 {
          tunnel: [TRUE ("Data Acquisition.Ready") FALSE ("Data Acquisition.Ready")] -> w329
          frame "ON", Default {
          }
          frame "OFF" {
          }
        }
        n118 = Bundle By Name(cluster=w330, "Data Acquisition.Ready"=w329) -> (w328:T1)
        n119 = call <vilib>:"Add State(s) to Queue__JKI_lib_State_Machine.vi"("State(s) in (\"\")"=w333) -> ("States Out"=w332:string)  [unwired: 14 in]
      }
      frame "System: Power Initialize" {
        # "Your code here.\n(You can make a copy of, or modify, this frame)"
        n120 = Unbundle By Name(w338) -> ("Data Acquisition.Setup.TempGrad"=w339:dbl)
        n121 = Equal To 0?(x=w339) -> (x = 0?=w336:bool)
        n122 = case shown="True" w336 {
          tunnel: ["UI: StatusString >> Enabling Relays\nArduino: Mode >> Cool\nUI: StatusString >> Enabling PSU output\nPSU: Mode >> ON" "UI: StatusString >> Enabling Relays\nArduino: Mode >> OFF\nUI: StatusString >> Enabling PSU output\nPSU: Mode >> OFF"] -> w337
          frame False {
            # "Standard Sample"
          }
          frame True {
            # "0 Gradient Sample"
          }
        }
        n123 = property on="Cooling label" class="Str"("Visible"=w336) -> ()  [unwired: 2 in, 2 out]
        n124 = call <vilib>:"Add State(s) to Queue__JKI_lib_State_Machine.vi"("State(s) in Front (\"\")"=w337, "State(s) in (\"\")"=w342) -> ("States Out"=w341:string)  [unwired: 13 in]
      }
      frame "System: Override" {
        # "Your code here.\n(You can make a copy of, or modify, this frame)"
        n125 = Bundle By Name(cluster=w348, "Data Acquisition.Ready"=TRUE ("System.Active")) -> (w347:T1)
        n126 = call <vilib>:"Add State(s) to Queue__JKI_lib_State_Machine.vi"("State(s) in Front (\"\")"="UI: Start Button >> Default\nUI: Temperature Buttons >> Show\nUI: RTM >> CDAQ_SHOW\nUI: RTM >> CAM_SHOW" ("State(s) in Front (\"\")"), "State(s) in (\"\")"=w351) -> ("States Out"=w350:string)  [unwired: 13 in]
      }
      frame "System: Stop" {
        # "Your code here.\n(You can make a copy of, or modify, this frame)"
        n127 = Unbundle By Name(w357) -> ("Manual Temp Control.Active"=w352:bool, "Data Acquisition.Active"=w354:bool)
        n128 = local write "Start"(FALSE ("Start")) -> ()
        n129 = Or(x=w352, y=w354) -> (x .or. y?=w353:bool)
        n130 = case shown="True" w353 {
          tunnel: w358 -> [_ w370]
          tunnel: w357 -> [w366 w369]
          tunnel: [w366 w368] -> w356
          tunnel: ["" ("State(s) in Front (\"\")") w367] -> w355
          frame False {
          }
          frame True {
            n131 = case shown="\"CPU_ERROR\"" w370 {
              tunnel: ["" ("State(s) in Front (\"\")") "UI: Alert >> Done" ("State(s) in Front (\"\")") "UI: Alert >> Process Overhead Error - Reduce Sample Size or Sample Rate \nUI: Start Button >> Error" ("State(s) in Front (\"\")") "UI: Alert >> Temperature Error, above maximum temperature!" ("State(s) in Front (\"\")")] -> w367
              tunnel: [w371 w373 w377 w379] -> w368
              tunnel: w369 -> [w371 w373 w378 w379]
              frame "False", Default {
              }
              frame "Done" {
              }
              frame "CPU_ERROR" {
                n132 = Bundle By Name(cluster=w378, "Data Acquisition.Ready"=FALSE) -> (w377:T1)
              }
              frame "TEMP_ERROR" {
              }
            }
          }
        }
        n133 = case shown="False" w354 {
          tunnel: [w383 "UI: Cursor Set >> Busy\nUI: StatusString >> Terminating Buffer\nData Acquisition: Buffer Terminate\nUI: StatusString >> Disabling Relays\nArduino: Mode >> OFF\nUI: StatusString >> Disabling PSU\nPSU: Mode >> OFF\nPSU: Output >> OFF\nUI: StatusString >> Unlocking files\nData: Files Unlock\nUI: StatusString >> Stamping Times\nData: Stamp times\nUI: Temperature Buttons >> Show\nUI: Time Left >> hide\nUI: StatusString >> Idle\nUI: Cursor Set >> Idle" ("State(s) in Front (\"\")")] -> w361
          tunnel: w356 -> [w381 w393]
          tunnel: [w382 w392] -> w360
          tunnel: w352 -> [w384 _]
          frame False {
            n134 = case shown="False" w384 {
              tunnel: ["UI: Cursor Set >> Busy\nUI: StatusString >> Disabling Relays\nArduino: Mode >> OFF\nUI: StatusString >> Disabling PSU\nPSU: Mode >> OFF\nPSU: Output >> OFF\nUI: Time Left >> hide\nUI: Temperature Buttons >> Show\nUI: StatusString >> Idle\nUI: Cursor Set >> Idle" ("State(s) in Front (\"\")") "UI: Cursor Set >> Busy\nUI: StatusString >> Disabling Relays\nArduino: Mode >> OFF\nUI: StatusString >> Disabling PSU\nPSU: Mode >> OFF\nPSU: Output >> OFF\nUI: Time Left >> hide\nUI: Temperature Buttons >> Show\nUI: StatusString >> Idle\nUI: Cursor Set >> Idle" ("State(s) in Front (\"\")")] -> w383
              tunnel: [w385 w388] -> w382
              tunnel: w381 -> [w385 w389]
              frame False {
              }
              frame True {
                n135 = Bundle By Name(cluster=w389, "Manual Temp Control.Active"=FALSE) -> (w388:T1)
              }
            }
          }
          frame True {
            n136 = Bundle By Name(cluster=w393, "Data Acquisition.Active"=FALSE ("System.Active")) -> (w392:T1)
          }
        }
        n137 = call <vilib>:"Add State(s) to Queue__JKI_lib_State_Machine.vi"("State(s) in Front (\"\")"=w361, "State(s) in (\"\")"=w364, "State(s) at Back (\"\")"=w355) -> ("States Out"=w363:string)  [unwired: 12 in]
      }
      frame "---------- Data ----------" {
        # "Do not put any code in this frame.\n(It is a separator no-op. You can make a copy of this frame to create a new Data frame)"
        n138 = call <vilib>:"Add State(s) to Queue__JKI_lib_State_Machine.vi"("State(s) in (\"\")"=w398) -> ("States Out"=w397:string)  [unwired: 14 in]
      }
      frame "Data: Initialize" {
        w408 = T11 {"Current VI Reference"=refnum, "Close Panel on Exit?"=FALSE, "Exit"=FALSE, "Initialized?"=FALSE}  # Core
        # "Initialize the shift-register data, here.\n(data names are defined by what you wire into the bundle function)"
        n139 = call "Settings_Load.vi"("error in"=w404) -> ("error out"=w405:errorcluster, "DataCluster out"=w406:T1)  [unwired: 9 in]
        n140 = call "Settings_Save.vi"("error in"=w405, "DataCluster"=w406) -> ("error out"=w403:errorcluster, "DataCluster dup"=w399:T1)  [unwired: 8 in]
        n141 = Unbundle By Name(T1 {"Core"={"Current VI Reference"=refnum, "Close Panel on Exit?"=FALSE, "Exit"=FALSE, "Initialized?"=FALSE}, "Connections"={"cDAQ"={"Task"="", "Connected"=FALSE, "Active"=FALSE, "ID"=""}, "Camera"={"Session"="", "Connected"=FALSE, "Active"=FALSE, "Placeholder"=refnum}, "PSU"={"Port"="", "Connected"=FALSE, "Active"=FALSE}, "Arduino"={"Port"="", "Connected"=FALSE, "Active"=FALSE}}, "Data Acquisition"={"Setup"={"Label"="", "Operator"="", "Notes"="", "TempGrad"=0.0, "TargetTemp"=0.0, "Sample Volume"=1.0}, "Camera"={"Image"=refnum, "Save Image"=refnum, "Image Frequency"=20, "Rectangle"={"Left"=0, "Top"=0, "Right"=0, "Bottom"=0, "Rotation"=0.0}, "Calibration"={"Top Left"={"X"=0.0, "Y"=0.0}, "Top Right"={"X"=0.0, "Y"=0.0}, "Bottom Left"={"X"=0.0, "Y"=0.0}, "Bottom Right"={"X"=0.0, "Y"=0.0}, "Fixpoint"={"X"=0.0, "Y"=0.0}, "Scan Area"=0.0, "Fixpoint Area"=0.0, "Well Pixels"=[], "Valid"=FALSE}, "FocusPos"=0, "Display Mapping"=10, "Camera Mode"=10}, "Thermistor"={"Sample Size"=0, "Calibration"={"B0.100"=[], "R25"=[], "c"=[], "State"=[], "V_S"=0.0, "R_S"=0.0}, "Timing Mode"=14713}, "Partition"={"Data"=[], "Cell Label"="", "Cell Color"=0, "Height"=10, "Width"=16, "Grid"=[]}, "Queue"={"Size"=0, "Queue"=refnum}, "Sample Rate"=0, "Active"=FALSE, "Ready"=FALSE, "Graph Mode"=0, "Gradient Buffer"=2}, "Control"={"Sample Rate"=0, "PID gains"={"proportional gain (Kc)"=0.0, "integral time (Ti, min)"=0.0, "derivative time (Td, min)"=0.0}}, "Manual Temp Control"={"TargetTemp"=1.0, "Mode"=0, "Active"=FALSE}} ("DataCluster")) -> ("Connections"=w400:T12)
        n142 = Bundle By Name(cluster=w399, "Core"=w408, "Connections"=w400, "Data Acquisition.Active"=FALSE ("System.Active")) -> (w409:T1)
        n143 = call <vilib>:"Add State(s) to Queue__JKI_lib_State_Machine.vi"("State(s) in Front (\"\")"="Data: Load Placeholder Image" ("State(s) in Front (\"\")"), "State(s) in (\"\")"=w411) -> ("States Out"=w410:string)  [unwired: 13 in]
      }
      frame "Data: Terminate" {
        # "Cleanup any data and references, here.\n(this is called automatically, by the Macro: Exit)"
        n144 = Bundle By Name(cluster=w417, "Data Acquisition.Camera.Calibration"=T8 {"Top Left"={"X"=0.0, "Y"=0.0}, "Top Right"={"X"=0.0, "Y"=0.0}, "Bottom Left"={"X"=0.0, "Y"=0.0}, "Bottom Right"={"X"=0.0, "Y"=0.0}, "Fixpoint"={"X"=0.0, "Y"=0.0}, "Scan Area"=0.0, "Fixpoint Area"=0.0, "Well Pixels"=[], "Valid"=FALSE}) -> (w413:T1)
        n145 = Unbundle By Name(w417) -> ("Core.Current VI Reference"=w418:refnum<vi>)
        n146 = call "Settings_Save.vi"("error in"=w416, "DataCluster"=w413) -> ("error out"=w415:errorcluster)  [unwired: 8 in, 1 out]
        n147 = Close Reference(reference=w418, error in (no error)=w415) -> (error out=w414:errorcluster)
        n148 = call <vilib>:"Add State(s) to Queue__JKI_lib_State_Machine.vi"("State(s) in (\"\")"=w420) -> ("States Out"=w419:string)  [unwired: 14 in]
      }
      frame "Data: Initialize Core Data" {
        # "Do not delete, rename, or modify this frame.\n(this is used to determine panel behavior on exit)"
        # "originally closed?"
        # "exe?"
        # "If panel starts closed or is an EXE, then close it when we exit"
        n149 = property class="VI"() -> ("FP.State"=w423:T7)  [unwired: 2 in, 2 out]
        n150 = property class="App"() -> ("App.Kind"=w429:T6)  [unwired: 2 in, 2 out]
        n151 = control-ref of="Current VI Reference"() -> (w424:refnum<vi>)
        n152 = Equal?(x=w423, y=T7."Closed" ("Front Panel Window:State")) -> (x = y?=w421:bool)
        n153 = Equal?(x=w429, y=T6."Run Time System" ("Application:Kind")) -> (x = y?=w427:bool)
        n154 = Or(x=w421, y=w427) -> (x .or. y?=w425:bool)
        n155 = Bundle By Name(cluster=w426, "Core.Current VI Reference"=w424, "Core.Close Panel on Exit?"=w425) -> (w431:T1)
        n156 = call <vilib>:"Add State(s) to Queue__JKI_lib_State_Machine.vi"("State(s) in (\"\")"=w433) -> ("States Out"=w432:string)  [unwired: 14 in]
      }
      frame "Data: Load Placeholder Image" {
        w440 = T13 4 items=["Grayscale (U8)", "Grayscale (I16)", "Grayscale (SGL)", "Complex (CSG)", "RGB (U32)", "HSL (U32)", "RGB (U64)", "Grayscale (U16)"] ("Image Type")
        # "Initialize the shift-register data, here.\n(data names are defined by what you wire into the bundle function)"
        n157 = call <vilib>:"Application Directory.vi"() -> ("Application Directory"=w444:path)
        n158 = Path To String(path=w444) -> (string=w446:string)
        n159 = call "IMAQ Create"("Image Name"="placeholder_img", "Image Type"=w440, "error in (no error)"=w436) -> ("New Image"=w443:T3, "error out"=w435:errorcluster)  [unwired: 2 in]
        n160 = Concatenate Strings(w446, "\\camera_placeholder.png") -> (w445:string)
        n161 = String To Path(string=w445) -> (path=w447:path)
        n162 = call "IMAQ ReadFile 2"("Use File Path Image Type"=FALSE, "File Path"=w447, "error in (no error)"=w435, "Image"=w443) -> ("error out"=w434:errorcluster, "Image Out"=w437:T3)  [unwired: 3 in, 3 out]
        n163 = local write "Camera Feed"(w437) -> ()
        n164 = Bundle By Name(cluster=w438, "Connections.Camera.Placeholder"=w437) -> (w448:T1)
        n165 = call <vilib>:"Add State(s) to Queue__JKI_lib_State_Machine.vi"("State(s) in (\"\")"=w450) -> ("States Out"=w449:string)  [unwired: 14 in]
      }
      frame "Data: Config" {
        # "Access Data Setup here.\n(this is called automatically, by the Settings Event Run time menu)"
        n166 = call "Settings_Config.vi"("DataCluster in"=w455) -> ("Canceled"=w452:bool, "DataCluster out"=w454:T1)  [unwired: 9 in]
        n167 = case shown="\"Start\"" w453 {
          tunnel: w452 -> [_ w463]
          tunnel: ["" w460] -> w451
          frame "False", Default {
          }
          frame "Start" {
            n168 = Select(t="System: Stop", s=w463, f="Data: Partition >> Start") -> (s? t:f=w460:string)
          }
        }
        n169 = call <vilib>:"Add State(s) to Queue__JKI_lib_State_Machine.vi"("State(s) in Front (\"\")"=w451, "State(s) in (\"\")"=w458) -> ("States Out"=w457:string)  [unwired: 13 in]
      }
      frame "Data: Partition" {
        # "Access Data Setup here.\n(this is called automatically, by the Settings Event Run time menu)"
        n170 = call "Partition_Setup.vi"("DataCluster in"=w468) -> ("Canceled?"=w465:bool, "DataCluster out"=w467:T1)  [unwired: 8 in, 1 out]
        n171 = case shown="\"Start\"" w466 {
          tunnel: w465 -> [_ w476]
          tunnel: ["" w473] -> w464
          frame "False", Default {
          }
          frame "Start" {
            n172 = Select(t="System: Stop", s=w476, f="System: Start") -> (s? t:f=w473:string)
          }
        }
        n173 = call <vilib>:"Add State(s) to Queue__JKI_lib_State_Machine.vi"("State(s) in Front (\"\")"=w464, "State(s) in (\"\")"=w471) -> ("States Out"=w470:string)  [unwired: 13 in]
      }
      frame "Data: Options" {
        # "Access Data Setup here.\n(this is called automatically, by the Settings Event Run time menu)"
        n174 = call "Options.vi"("DataCluster in"=w480) -> ("State"=w478:string, "DataCluster out"=w479:T1)  [unwired: 9 in]
        n175 = call <vilib>:"Add State(s) to Queue__JKI_lib_State_Machine.vi"("State(s) in Front (\"\")"=w478, "State(s) in (\"\")"=w482) -> ("States Out"=w481:string)  [unwired: 13 in]
      }
      frame "Data: Calibration" {
        # "Access Data Setup here.\n(this is called automatically, by the Settings Event Run time menu)"
        n176 = call "Thermistor_Callibration.vi"("DataCluster in"=w485) -> ("State Out"=w483:string, "DataCluster out"=w484:T1)  [unwired: 9 in]
        n177 = call <vilib>:"Add State(s) to Queue__JKI_lib_State_Machine.vi"("State(s) in Front (\"\")"=w483, "State(s) in (\"\")"=w488) -> ("States Out"=w487:string)  [unwired: 13 in]
      }
      frame "Data: Load Calibration" {
        # "Access Data Setup here.\n(this is called automatically, by the Settings Event Run time menu)"
        n178 = call "Thermistor_Callibration_Load.vi"("error in"=w491, "DataCluster"=w493) -> ("error out"=w490:errorcluster, "State"=w489:string, "DataCluster out"=w492:T1)  [unwired: 7 in]
        n179 = call <vilib>:"Add State(s) to Queue__JKI_lib_State_Machine.vi"("State(s) in Front (\"\")"=w489, "State(s) in (\"\")"=w495) -> ("States Out"=w494:string)  [unwired: 13 in]
      }
      frame "Data: Load Thermal Calibration" {
        # "Access Data Setup here.\n(this is called automatically, by the Settings Event Run time menu)"
        n180 = call "TCam_CalibrationLoad.vi"("error in (no error)"=w498, "DataCluster"=w500) -> ("error out"=w497:errorcluster, "state out"=w496:string, "output cluster"=w499:T1)  [unwired: 7 in]
        n181 = call <vilib>:"Add State(s) to Queue__JKI_lib_State_Machine.vi"("State(s) in Front (\"\")"=w496, "State(s) in (\"\")"=w502) -> ("States Out"=w501:string)  [unwired: 13 in]
      }
      frame "Data: Calculate Wells" {
        w504 = u16 0 items=["384 (24x16)", "96 (12x8)"] ("Size")
        # "Access Data Setup here.\n(this is called automatically, by the Settings Event Run time menu)"
        n182 = call "TCam_WellPixels.vi"("Size"=w504, "DataCluster"=w507) -> ("output cluster"=w506:T1)  [unwired: 9 in]
        n183 = call <vilib>:"Add State(s) to Queue__JKI_lib_State_Machine.vi"("State(s) in (\"\")"=w505) -> ("States Out"=w508:string)  [unwired: 14 in]
      }
      frame "Data: Save Calibration" {
        # "Access Data Setup here.\n(this is called automatically, by the Settings Event Run time menu)"
        n184 = call "Thermistor_Callibration_Save.vi"("error in"=w511, "DataCluster"=w509) -> ("error out"=w510:errorcluster)  [unwired: 9 in]
        n185 = call <vilib>:"Add State(s) to Queue__JKI_lib_State_Machine.vi"("State(s) in (\"\")"=w513) -> ("States Out"=w512:string)  [unwired: 14 in]
      }
      frame "Data: Setup File Config" {
        # "Access Data Setup here.\n(this is called automatically, by the Settings Event Run time menu)"
        n186 = call "SetupFile_Create.vi"("error in (no error)"=w516, "DataCluster"=w517) -> ("error out"=w515:errorcluster, "DataCluster out"=w514:T1)  [unwired: 8 in]
        n187 = call <vilib>:"Add State(s) to Queue__JKI_lib_State_Machine.vi"("State(s) in (\"\")"=w519) -> ("States Out"=w518:string)  [unwired: 14 in]
      }
      frame "Data: Data File Config" {
        # "Access Data Setup here.\n(this is called automatically, by the Settings Event Run time menu)"
        n188 = call "DataFile_Create.vi"("error in (no error)"=w521, "DataCluster"=w522) -> ("error out"=w520:errorcluster)  [unwired: 9 in]
        n189 = call <vilib>:"Add State(s) to Queue__JKI_lib_State_Machine.vi"("State(s) in (\"\")"=w524) -> ("States Out"=w523:string)  [unwired: 14 in]
      }
      frame "Data: Files Unlock" {
        # "Access Data Setup here.\n(this is called automatically, by the Settings Event Run time menu)"
        n190 = Unbundle By Name(w534) -> ("Data Acquisition.Setup.Label"=w542:string)
        n191 = call <vilib>:"Application Directory.vi"() -> ("Application Directory"=w540:path)
        n192 = Path To String(path=w540) -> (string=w541:string)
        n193 = Concatenate Strings(w541, "\\Data\\", w542) -> (w527:string)
        n194 = Concatenate Strings(w527, "\\Partition.csv") -> (w530:string)
        n195 = Concatenate Strings(w527, "\\Setup.csv") -> (w544:string)
        n196 = Concatenate Strings(w527, "\\Data.csv") -> (w543:string)
        n197 = String To Path(string=w530) -> (path=w531:path)
        n198 = String To Path(string=w544) -> (path=w545:path)
        n199 = String To Path(string=w543) -> (path=w546:path)
        n200 = Set Permissions(7:i16 448 ("permissions"), 8:w526, 11:w531) -> (0:w525:errorcluster)  [unwired: 2 in, 1 out]
        n201 = Set Permissions(7:i16 448 ("permissions"), 8:w525, 11:w546) -> (0:w533:errorcluster)  [unwired: 2 in, 1 out]
        n202 = Set Permissions(7:i16 448 ("permissions"), 8:w533, 11:w545) -> (0:w532:errorcluster)  [unwired: 2 in, 1 out]
        n203 = call <vilib>:"Add State(s) to Queue__JKI_lib_State_Machine.vi"("State(s) in (\"\")"=w548) -> ("States Out"=w547:string)  [unwired: 14 in]
      }
      frame "Data: Stamp times" {
        # "Access Data Setup here.\n(this is called automatically, by the Settings Event Run time menu)"
        n204 = call "SetupFile_Stamp.vi"("error in (no error)"=w551, "DataCluster"=w550) -> ("error out"=w552:errorcluster, "DataCluster out"=w549:T1)  [unwired: 8 in]
        n205 = call <vilib>:"Add State(s) to Queue__JKI_lib_State_Machine.vi"("State(s) in (\"\")"=w554) -> ("States Out"=w553:string)  [unwired: 14 in]
      }
      frame "Data: Open Folder" {
        # "Access Data Setup here.\n(this is called automatically, by the Settings Event Run time menu)"
        n206 = Unbundle By Name(w562) -> ("Data Acquisition.Setup.Label"=w566:string)
        n207 = call <vilib>:"Application Directory.vi"() -> ("Application Directory"=w564:path)
        n208 = Path To String(path=w564) -> (string=w565:string)
        n209 = Concatenate Strings(w565, "\\Data\\", w566) -> (w561:string)
        n210 = String To Path(string=w561) -> (path=w559:path)
        n211 = Format Into String(format string="cmd /c explorer.exe \"%s\"", w559) -> (resulting string=w558:string)  [unwired: 2 in, 1 out]
        n212 = call <vilib>:"System Exec.vi"("run minimized? (F)"=TRUE, "error in (no error)"=w556, "command line"=w558) -> ("error out"=w555:errorcluster)  [unwired: 5 in, 3 out]
        n213 = call <vilib>:"Add State(s) to Queue__JKI_lib_State_Machine.vi"("State(s) in (\"\")"=w568) -> ("States Out"=w567:string)  [unwired: 14 in]
      }
      frame "Data: Image Folder Setup" {
        # "Access Data Setup here.\n(this is called automatically, by the Settings Event Run time menu)"
        n214 = Unbundle By Name(w572) -> ("Data Acquisition.Setup.Label"=w574:string)
        n215 = call <vilib>:"Application Directory.vi"() -> ("Application Directory"=w581:path)
        n216 = Path To String(path=w581) -> (string=w580:string)
        n217 = Concatenate Strings(w580, "\\Data\\", w574, "\\Images\\" ("string")) -> (w578:string)
        n218 = String To Path(string=w578) -> (path=w577:path)
        n219 = call <vilib>:"Check if File or Folder Exists.vi"("error in (no error)"=w571, "path"=w577) -> ("error out"=w573:errorcluster, "file or folder exists?"=w576:bool, "dup path"=w575:path)  [unwired: 7 in]
        n220 = case shown="False" w576 {
          tunnel: w575 -> [w586 _]
          tunnel: w573 -> [w585 w587]
          tunnel: [w584 w587] -> w570
          frame False {
            n221 = Create Folder(path (use dialog)=w586, error in=w585) -> (error out=w584:errorcluster)  [unwired: 1 in, 2 out]
          }
          frame True {
          }
        }
        n222 = call <vilib>:"Add State(s) to Queue__JKI_lib_State_Machine.vi"("State(s) in (\"\")"=w583) -> ("States Out"=w582:string)  [unwired: 14 in]
      }
      frame "---------- Connections ----------" {
        # "Do not put any code in this frame.\n(It is a separator no-op. You can make a copy of this frame to create a new Data frame)"
        n223 = call <vilib>:"Add State(s) to Queue__JKI_lib_State_Machine.vi"("State(s) in (\"\")"=w591) -> ("States Out"=w590:string)  [unwired: 14 in]
      }
      frame "Connections: Initialize" {
        # "Initialize the System Connections, here.\n(this is called automatically, by the Macro: Init)"
        n224 = call <vilib>:"Add State(s) to Queue__JKI_lib_State_Machine.vi"("State(s) in Front (\"\")"="UI: StatusString >> Scanning for cDAQ\ncDAQ: Scan\nLoading UI: Progress\nUI: StatusString >> Connecting cDAQ (Thermistors)\ncDAQ: Initialize\nLoading UI: Progress\nUI: StatusString >> Connecting Camera\nCamera: Initialize\nLoading UI: Progress\nUI: StatusString >> Connecting MCU\nArduino: Initialize\nLoading UI: Progress\nUI: StatusString >> Connecting Power Supply\nPSU: Initialize\nLoading UI: Progress\nUI: StatusString >> Validating Connections\nConnections: Status\nLoading UI: Progress\n// ----------- Data Acquisition Setup----------- //\nUI: StatusString >> Initializing cDAQ\nData Acquisition: cDAQ Initialize\nLoading UI: Progress\nUI: StatusString >> Initializing Camera\nData Acquisition: Camera Initialize\nLoading UI: Progress\nUI: Chart Clear\nUI: Chart Setup\nUI: Cursor Set >> Idle\nUI: StatusString >> Idle" ("State(s) in Front (\"\")"), "State(s) in (\"\")"=w596) -> ("States Out"=w595:string)  [unwired: 13 in]
      }
      frame "Connections: Terminate" {
        # "Terminate connection to DAQs and Power Supply (Peltier)"
        # "Terminate the System Connections, here.\n(this is called automatically, by the Macro: Exit)"
        n225 = Bundle By Name(cluster=w602, "Data Acquisition.Ready"=FALSE) -> (w598:T1)
        n226 = call "Stall Data Flow.vim"("value in"="UI: StatusString >> Terminating cDAQ Connection\ncDAQ: Terminate\nUI: StatusString >> Terminating Camera Connection\nCamera: Terminate\nUI: StatusString >> Terminating Power Supply\nPSU: Mode >> OFF\nPSU: Terminate" ("State(s) in Front (\"\")"), "milliseconds to wait"=u32 250) -> ("value out"=w600:string)  [unwired: 1 out]
        n227 = call <vilib>:"Add State(s) to Queue__JKI_lib_State_Machine.vi"("State(s) in Front (\"\")"=w600, "State(s) in (\"\")"=w605) -> ("States Out"=w604:string)  [unwired: 13 in]
      }
      frame "Connections: Status" {
        # "Checks Connection Status , here.\n(this is called automatically, by the Connections: Initialize)"
        n228 = Unbundle By Name(w610) -> ("Connections.cDAQ.Connected"=w612:bool, "Connections.Camera.Connected"=w608:bool, "Connections.PSU.Connected"=w607:bool, "Connections.Arduino.Connected"=w606:bool)
        n229 = Compound Arithmetic op=AND(w612, w608, w607, w606) -> (w613:bool)
        n230 = case shown="False" w613 {
          selector: w613 -> [w617 w621]
          tunnel: ["UI: Start Button >> Error\nUI: Temperature Buttons >> Hide\nUI: StatusString >> Connection Error!" "Loading UI: Description >> Connections Successful\nUI: Start Button >> Default\nUI: Temperature Buttons >> Show\nUI: StatusString >> Idle"] -> w611
          tunnel: w610 -> [w619 w623]
          tunnel: [w618 w622] -> w609
          frame False {
            n231 = Bundle By Name(cluster=w619, "Data Acquisition.Ready"=w617) -> (w618:T1)
          }
          frame True {
            n232 = Bundle By Name(cluster=w623, "Data Acquisition.Ready"=w621) -> (w622:T1)
          }
        }
        n233 = call <vilib>:"Add State(s) to Queue__JKI_lib_State_Machine.vi"("State(s) in Front (\"\")"=w611, "State(s) in (\"\")"=w616) -> ("States Out"=w615:string)  [unwired: 13 in]
      }
      frame "---------- UI ----------" {
        # "Do not put any code in this frame.\n(It is a separator no-op. You can make a copy of this frame to create a new UI frame)"
        n234 = call <vilib>:"Add State(s) to Queue__JKI_lib_State_Machine.vi"("State(s) in (\"\")"=w628) -> ("States Out"=w627:string)  [unwired: 14 in]
      }
      frame "UI: Initialize" {
        w634 = u32[] [] ("History Data")
        w629 = FALSE ("Visible")
        # "Initialize the User Interface, here.\n(this is called automatically, by the Macro: Init)"
        n235 = control-ref of="This VI"() -> (w635:refnum<vi>)
        n236 = property on="DP_Overhead" class="WFChart (strict)"("Visible"=w629) -> ()  [unwired: 2 in, 2 out]
        n237 = property on="cDAQ_Time" class="WFChart (strict)"("Visible"=w629) -> ()  [unwired: 2 in, 2 out]
        n238 = property on="DL_Time" class="WFChart (strict)"("Visible"=w629) -> ()  [unwired: 2 in, 2 out]
        n239 = property class="VI" props=["Clone Name"](reference=w635) -> ()  [unwired: 1 in, 3 out]
        n240 = property on="Error Array" class="Arr (strict)"("Visible"=w629) -> ()  [unwired: 2 in, 2 out]
        n241 = property on="Cooling label" class="Str"("Visible"=w629) -> ()  [unwired: 2 in, 2 out]
        n242 = local write "OverlayTemp?"(FALSE ("Display?")) -> ()
        n243 = local write "Start"(FALSE ("Start")) -> ()
        n244 = local write "Error Array"(errorcluster[] [] ("Error Array")) -> ()
        n245 = property on="DL_Time" class="WFChart (strict)"("History Data"=w634) -> ()  [unwired: 2 in, 2 out]
        n246 = property on="DP_Overhead" class="WFChart (strict)"("History Data"=w634) -> ()  [unwired: 2 in, 2 out]
        n247 = call <vilib>:"Add State(s) to Queue__JKI_lib_State_Machine.vi"("State(s) in Front (\"\")"="UI: StatusString >> Clearing Chart History\nUI: Chart Setup\nUI: Chart Clear\nUI: Image Setup\nUI: Time Left >> hide\nUI: Temperature Buttons >> Hide" ("State(s) in Front (\"\")"), "State(s) in (\"\")"=w642) -> ("States Out"=w641:string)  [unwired: 13 in]
        "Title" <- "Ice Nucleation Contoller" ("Version")
        "Galium Control" <- "Galium Control" ("Galium Control")
        "Cooling label" <- "Cooling Disabled!" ("Cooling label")
      }
      frame "UI: StatusString" {
        # "Argument"
        # "Set Status String here\n(this is called takes argument and applies to Status String)"
        n248 = call <vilib>:"Add State(s) to Queue__JKI_lib_State_Machine.vi"("State(s) in (\"\")"=w647) -> ("States Out"=w646:string)  [unwired: 14 in]
        "StatusString" <- w643
      }
      frame "UI: Chart Setup" {
        # "Initialize the User Interface, here.\n(this is called automatically, by the Macro: Init)"
        n249 = property on="Temps" class="WFChart (strict)"("XScale.Maximum"=300.0 ("X Scale.Range:Maximum"), "XScale.Minimum"=0.0 ("X Scale.Range:Minimum"), "ActYScl"=0 ("Active Y Scale"), "YScale.Maximum"=50.0 ("X Scale.Range:Maximum"), "YScale.Minimum"=-40.0 ("X Scale.Range:Minimum")) -> ()  [unwired: 2 in, 2 out]
        n250 = property on="Gradients" class="WFChart (strict)"("XScale.Maximum"=300.0 ("X Scale.Range:Maximum"), "XScale.Minimum"=0.0 ("X Scale.Range:Minimum"), "ActYScl"=0 ("Active Y Scale"), "YScale.Maximum"=2.0 ("Y Scale.Range:Maximum"), "YScale.Minimum"=-2.0 ("Y Scale.Range:Minimum")) -> ()  [unwired: 2 in, 2 out]
        n251 = call <vilib>:"Add State(s) to Queue__JKI_lib_State_Machine.vi"("State(s) in (\"\")"=w661) -> ("States Out"=w660:string)  [unwired: 14 in]
      }
      frame "UI: Chart Clear" {
        (unwired) TRUE
        w662 = waveform(dbl)[][] [] ("History Data")
        # "Initialize the User Interface, here.\n(this is called automatically, by the Macro: Init)"
        n252 = property on="Temps" class="WFChart (strict)"("History Data"=w662) -> ()  [unwired: 2 in, 2 out]
        n253 = property on="Gradients" class="WFChart (strict)"("History Data"=w662) -> ()  [unwired: 2 in, 2 out]
        n254 = call <vilib>:"Add State(s) to Queue__JKI_lib_State_Machine.vi"("State(s) in (\"\")"=w666) -> ("States Out"=w665:string)  [unwired: 14 in]
      }
      frame "UI: Time Left" {
        # "Initialize the User Interface, here.\n(this is called automatically, by the Macro: Init)"
        n255 = case shown="\"hide\", Default" w668 {
          tunnel: [FALSE TRUE] -> w667
          frame "hide", Default {
          }
          frame "show" {
          }
        }
        n256 = property on="T_Left" class="Str"("Visible"=w667) -> ()  [unwired: 2 in, 2 out]
        n257 = call <vilib>:"Add State(s) to Queue__JKI_lib_State_Machine.vi"("State(s) in (\"\")"=w672) -> ("States Out"=w671:string)  [unwired: 14 in]
      }
      frame "UI: Image Setup" {
        # "Initialize the User Interface, here.\n(this is called automatically, by the Macro: Init)"
        n258 = Unbundle By Name(w675) -> ("Data Acquisition.Camera.Display Mapping"=w676:u32)
        n259 = property on="Camera Feed" class="ImageControl"("16-bit Display Conversion Method"=w676) -> ()  [unwired: 2 in, 2 out]
        n260 = call <vilib>:"Add State(s) to Queue__JKI_lib_State_Machine.vi"("State(s) in (\"\")"=w679) -> ("States Out"=w678:string)  [unwired: 14 in]
      }
      frame "UI: Help" {
        # "Argument"
        # "Set Status String here\n(this is called takes argument and applies to Status String)"
        n261 = case shown="\"About\"" w680 {
          frame "False", Default {
          }
          frame "About" {
            n262 = call "Read Exe Version.vi"("Application name"=path "INC.exe") -> ("String"=w686:string)  [unwired: 7 in, 3 out]
            n263 = Concatenate Strings("Ice Nucleation Control Software\n\n" ("message"), w686) -> (w687:string)
            n264 = One Button Dialog(message=w687) -> ()  [unwired: 1 in, 1 out]
          }
        }
        n265 = call <vilib>:"Add State(s) to Queue__JKI_lib_State_Machine.vi"("State(s) in (\"\")"=w684) -> ("States Out"=w683:string)  [unwired: 14 in]
      }
      frame "UI: Popup" {
        # "Argument"
        # "Set Status String here\n(this is called takes argument and applies to Status String)"
        n266 = One Button Dialog(message=w689) -> ()  [unwired: 1 in, 1 out]
        n267 = call <vilib>:"Add State(s) to Queue__JKI_lib_State_Machine.vi"("State(s) in (\"\")"=w693) -> ("States Out"=w692:string)  [unwired: 14 in]
      }
      frame "UI: Alert" {
        # "Argument"
        # "Set Status String here\n(this is called takes argument and applies to Status String)"
        n268 = case shown="\"Done\"" w694 {
          selector: w694 -> [_ w700]
          frame "Done" {
            n269 = call <vilib>:"Beep.vi"() -> ()  [unwired: 12 in]
            n270 = One Button Dialog(message="Target temperature reached") -> ()  [unwired: 1 in, 1 out]
          }
          frame Default {
            n271 = call <vilib>:"Beep.vi"() -> ()  [unwired: 12 in]
            n272 = One Button Dialog(message=w700) -> ()  [unwired: 1 in, 1 out]
          }
        }
        n273 = call <vilib>:"Add State(s) to Queue__JKI_lib_State_Machine.vi"("State(s) in (\"\")"=w698) -> ("States Out"=w697:string)  [unwired: 14 in]
      }
      frame "UI: Connections Status" {
        # "Set Status String here\n(this is called takes argument and applies to Status String)"
        n274 = Unbundle By Name(w706) -> ("Connections.cDAQ.Connected"=w705:bool, "Connections.Camera.Connected"=w704:bool, "Connections.PSU.Connected"=w702:bool, "Connections.Arduino.Connected"=w701:bool)
        n275 = call "ConnectionStatus.vi"("MCU_status"=w701, "PSU_status"=w702, "Camera_status"=w704, "cDAQ_Therm_status"=w705) -> ("String"=w703:string)  [unwired: 6 in, 1 out]
        n276 = call <vilib>:"Add State(s) to Queue__JKI_lib_State_Machine.vi"("State(s) in Front (\"\")"=w703, "State(s) in (\"\")"=w709) -> ("States Out"=w708:string)  [unwired: 13 in]
      }
      frame "UI: Start Button" {
        # "Argument"
        # "Set Status String here\n(this is called takes argument and applies to Status String)"
        n277 = case shown="\"Error\"" w712 {
          tunnel: [cluster{u32, u32}[] [{8388608, 8388608}, {4367360, 4367360}, {9342611, 9342611}, {6710891, 6710891}, {16711681, 16711680}, {16711681, 16711680}] ("Colors [4]") cluster{u32, u32}[] [{4367360, 12369084}, {10621999, 10621999}, {10621999, 10621999}, {4367360, 1985280}, {4367360, 1985280}, {10621999, 10621999}] ("Colors [4]") cluster{u32, u32}[] [{1985280, 12369084}, {4367360, 4367360}, {8388608, 16711681}, {1985280, 1985280}, {1985280, 4367360}, {8388608, 16711681}] ("Colors [4]")] -> _
          tunnel: [string[] ["Error", "Error", "Error", "Error"] ("Strings [4]") string[] ["Start", "Stop", "Stop", "Start"] ("Strings [4]") string[] ["Connecting", "Connecting", "Connecting", "Connecting"] ("Strings [4]")] -> w711
          tunnel: [T9."Enabled" ("Disabled") T9."Enabled" ("Disabled") T9."Disabled" ("Disabled")] -> w710
          frame "Error" {
          }
          frame "Default", Default {
          }
          frame "Connecting" {
          }
        }
        n278 = property on="Start" class="Bool (strict)"("Strings [4]"=w711, "DisabledEnum"=w710) -> ()  [unwired: 2 in, 2 out]
        n279 = call <vilib>:"Add State(s) to Queue__JKI_lib_State_Machine.vi"("State(s) in (\"\")"=w716) -> ("States Out"=w715:string)  [unwired: 14 in]
      }
      frame "UI: Temperature Buttons" {
        # "Argument"
        # "Set Status String here\n(this is called takes argument and applies to Status String)"
        n280 = Unbundle By Name(w728) -> ("Data Acquisition.Ready"=w727:bool)
        n281 = case shown="\"Show\"" w730 {
          tunnel: [w734 w735] -> w729
          tunnel: [w734 w735] -> w726
          tunnel: w727 -> [_ _]
          frame "Hide", Default {
            w734 = FALSE
          }
          frame "Show" {
            w735 = TRUE
          }
        }
        n282 = property on="Freeze" class="Bool"("Visible"=w726) -> ()  [unwired: 2 in, 2 out]
        n283 = property on="Galium Control" class="Str"("Visible"=w726) -> ()  [unwired: 2 in, 2 out]
        n284 = property on="Melt" class="Bool"("Visible"=w729) -> ()  [unwired: 2 in, 2 out]
        n285 = call <vilib>:"Add State(s) to Queue__JKI_lib_State_Machine.vi"("State(s) in (\"\")"=w733) -> ("States Out"=w732:string)  [unwired: 14 in]
      }
      frame "UI: RTM" {
        # "Argument"
        # "Set Status String here\n(this is called takes argument and applies to Status String)"
        n286 = Current VI's Menubar() -> (w736:refnum<k9>)
        n287 = case shown="\"CAM_HIDE\"" w737 {
          tunnel: w736 -> [w745 w749 w752 w755 w756 w761 _ _]
          frame "CAM_SHOW" {
            n288 = Set Menu Item Info(7:"MENU_CAM" ("item name"), 9:TRUE ("enabled"), 11:w745) -> ()  [unwired: 4 in, 2 out]
            n289 = property on="Camera Feed" class="ImageControl"("DisabledEnum"=T9."Enabled" ("Disabled")) -> ()  [unwired: 2 in, 2 out]
          }
          frame "CAM_HIDE" {
            n290 = Set Menu Item Info(7:"MENU_CAM" ("item name"), 9:FALSE ("enabled"), 11:w749) -> ()  [unwired: 4 in, 2 out]
            n291 = property on="Camera Feed" class="ImageControl"("DisabledEnum"=T9."Disabled and Grayed Out" ("Disabled")) -> ()  [unwired: 2 in, 2 out]
          }
          frame "CDAQ_HIDE" {
            n292 = Set Menu Item Info(7:"MENU_CDAQ" ("item name"), 9:FALSE ("enabled"), 11:w752) -> ()  [unwired: 4 in, 2 out]
          }
          frame "CDAQ_SHOW" {
            n293 = Set Menu Item Info(7:"MENU_CDAQ" ("item name"), 9:TRUE ("enabled"), 11:w755) -> ()  [unwired: 4 in, 2 out]
          }
          frame "TEMP_SHOW" {
            n294 = Set Menu Item Info(7:"TEMP_MELT" ("item name"), 9:TRUE ("enabled"), 11:w756) -> ()  [unwired: 4 in, 2 out]
            n295 = Set Menu Item Info(7:"TEMP_FREEZE" ("item name"), 9:TRUE ("enabled"), 11:w756) -> ()  [unwired: 4 in, 2 out]
          }
          frame "TEMP_HIDE" {
            n296 = Set Menu Item Info(7:"TEMP_MELT" ("item name"), 9:FALSE ("enabled"), 11:w761) -> ()  [unwired: 4 in, 2 out]
            n297 = Set Menu Item Info(7:"TEMP_FREEZE" ("item name"), 9:FALSE ("enabled"), 11:w761) -> ()  [unwired: 4 in, 2 out]
          }
          frame "Default", Default {
          }
          frame "Connecting" {
          }
        }
        n298 = call <vilib>:"Add State(s) to Queue__JKI_lib_State_Machine.vi"("State(s) in (\"\")"=w741) -> ("States Out"=w740:string)  [unwired: 14 in]
      }
      frame "UI: Cursor Set" {
        # "Argument"
        # "Set and Unset Cursor Busy.\n(Usage: \"UI: Cursor Set >> Busy|Idle\")"
        n299 = case shown="\"Idle\", Default" w766 {
          tunnel: w768 -> [w773 w775]
          tunnel: [w772 w774] -> w767
          frame "Idle", Default {
            n300 = call <vilib>:"Unset Busy.vi"("error in (no error)"=w773) -> ("error out"=w772:errorcluster)  [unwired: 10 in]
          }
          frame "Busy" {
            n301 = call <vilib>:"Set Busy.vi"("error in (no error)"=w775) -> ("error out"=w774:errorcluster)  [unwired: 9 in, 1 out]
          }
        }
        n302 = call <vilib>:"Add State(s) to Queue__JKI_lib_State_Machine.vi"("State(s) in (\"\")"=w771) -> ("States Out"=w770:string)  [unwired: 14 in]
      }
      frame "UI: Front Panel State" {
        # "Argument"
        # "Set Front Panel Open or Closed\n(Usage: \"UI: Front Panel State >> Open|Close\")"
        n303 = Unbundle By Name(w778) -> ("Core.Current VI Reference"=w777:refnum<vi>)
        n304 = case shown="\"Open\", \"Standard\", Default" w776 {
          tunnel: w780 -> [w788 w803 w814 w827 w840]
          tunnel: [w790 w804 w816 w829 w842] -> w779
          tunnel: w777 -> [w789 w801 w815 w828 w841]
          frame "Open", "Standard", Default {
            w783 = T7."Standard" ("State")
            n305 = property class="VI"(reference=w789, error in=w788) -> (reference out=w786:refnum<vi>, error out=w787:errorcluster, "FP.State"=w785:T7)
            n306 = Not Equal?(x=w785, y=w783) -> (x != y?=w784:bool)
            n307 = case shown="True" w784 {
              tunnel: [w794 w796] -> w790
              tunnel: w787 -> [w793 w796]
              tunnel: w786 -> [w792 _]
              tunnel: w783 -> [w791 _]
              frame True {
                n308 = invoke class="VI" method="FP.Open"(reference=w792, error in=w793, "Activate"=TRUE, "State"=w791) -> (error out=w794:errorcluster)  [unwired: 1 in, 4 out]
              }
              frame False {
              }
            }
          }
          frame "Close", "Closed" {
            n309 = property class="VI"(reference=w801, error in=w803) -> (reference out=w800:refnum<vi>, error out=w802:errorcluster, "FP.State"=w798:T7)
            n310 = Not Equal?(x=w798, y=T7."Closed" ("Front Panel Window:State")) -> (x != y?=w797:bool)
            n311 = case shown="True" w797 {
              tunnel: [w805 w808] -> w804
              tunnel: w802 -> [w805 w807]
              tunnel: w800 -> [_ w806]
              frame False {
              }
              frame True {
                n312 = invoke class="VI" method="FP.Close"(reference=w806, error in=w807) -> (error out=w808:errorcluster)  [unwired: 1 in, 2 out]
              }
            }
          }
          frame "Hidden", "Hide" {
            w809 = T7."Hidden" ("State")
            n313 = property class="VI"(reference=w815, error in=w814) -> (reference out=w812:refnum<vi>, error out=w813:errorcluster, "FP.State"=w811:T7)
            n314 = Not Equal?(x=w811, y=w809) -> (x != y?=w810:bool)
            n315 = case shown="True" w810 {
              tunnel: [w820 w821] -> w816
              tunnel: w813 -> [w819 w821]
              tunnel: w812 -> [w818 _]
              tunnel: w809 -> [w817 _]
              frame True {
                n316 = invoke class="VI" method="FP.Open"(reference=w818, error in=w819, "State"=w817) -> (error out=w820:errorcluster)  [unwired: 2 in, 4 out]
              }
              frame False {
              }
            }
          }
          frame "Minimize", "Minimized" {
            w822 = T7."Minimized" ("State")
            n317 = property class="VI"(reference=w828, error in=w827) -> (reference out=w825:refnum<vi>, error out=w826:errorcluster, "FP.State"=w824:T7)
            n318 = Not Equal?(x=w824, y=w822) -> (x != y?=w823:bool)
            n319 = case shown="True" w823 {
              tunnel: [w833 w834] -> w829
              tunnel: w826 -> [w832 w834]
              tunnel: w825 -> [w831 _]
              tunnel: w822 -> [w830 _]
              frame True {
                n320 = invoke class="VI" method="FP.Open"(reference=w831, error in=w832, "State"=w830) -> (error out=w833:errorcluster)  [unwired: 2 in, 4 out]
              }
              frame False {
              }
            }
          }
          frame "Maximize", "Maximized" {
            w835 = T7."Maximized" ("State")
            n321 = property class="VI"(reference=w841, error in=w840) -> (reference out=w838:refnum<vi>, error out=w839:errorcluster, "FP.State"=w837:T7)
            n322 = Not Equal?(x=w837, y=w835) -> (x != y?=w836:bool)
            n323 = case shown="True" w836 {
              tunnel: [w846 w847] -> w842
              tunnel: w839 -> [w845 w847]
              tunnel: w838 -> [w844 _]
              tunnel: w835 -> [w843 _]
              frame True {
                n324 = invoke class="VI" method="FP.Open"(reference=w844, error in=w845, "State"=w843) -> (error out=w846:errorcluster)  [unwired: 2 in, 4 out]
              }
              frame False {
              }
            }
          }
        }
        n325 = call <vilib>:"Add State(s) to Queue__JKI_lib_State_Machine.vi"("State(s) in (\"\")"=w782) -> ("States Out"=w781:string)  [unwired: 14 in]
      }
      frame "---------- Loading UI ----------" {
        # "Do not put any code in this frame.\n(It is a separator no-op. You can make a copy of this frame to create a new UI frame)"
        n326 = call <vilib>:"Add State(s) to Queue__JKI_lib_State_Machine.vi"("State(s) in (\"\")"=w851) -> ("States Out"=w850:string)  [unwired: 14 in]
      }
      frame "Loading UI: Exit" {
        # "Do not put any code in this frame.\n(It is a separator no-op. You can make a copy of this frame to create a new UI frame)"
        n327 = Bundle By Name(cluster=w854, "Core.Initialized?"=TRUE) -> (w853:T1)
        n328 = call <vilib>:"Add State(s) to Queue__JKI_lib_State_Machine.vi"("State(s) in (\"\")"=w857) -> ("States Out"=w856:string)  [unwired: 14 in]
      }
      frame "Loading UI: Description" {
        # "Do not put any code in this frame.\n(It is a separator no-op. You can make a copy of this frame to create a new UI frame)"
        n329 = call <vilib>:"Add State(s) to Queue__JKI_lib_State_Machine.vi"("State(s) in (\"\")"=w861) -> ("States Out"=w860:string)  [unwired: 14 in]
      }
      frame "Loading UI: Progress" {
        # "Do not put any code in this frame.\n(It is a separator no-op. You can make a copy of this frame to create a new UI frame)"
        n330 = call <vilib>:"Add State(s) to Queue__JKI_lib_State_Machine.vi"("State(s) in (\"\")"=w865) -> ("States Out"=w864:string)  [unwired: 14 in]
      }
      frame "Loading UI: Version" {
        # "Do not put any code in this frame.\n(It is a separator no-op. You can make a copy of this frame to create a new UI frame)"
        n331 = call <vilib>:"Add State(s) to Queue__JKI_lib_State_Machine.vi"("State(s) in (\"\")"=w869) -> ("States Out"=w868:string)  [unwired: 14 in]
      }
      frame "Loading UI: Initialize" {
        # "Do not put any code in this frame.\n(It is a separator no-op. You can make a copy of this frame to create a new UI frame)"
        n332 = Bundle By Name(cluster=w873, "Core.Initialized?"=FALSE) -> (w872:T1)
        n333 = call <vilib>:"Add State(s) to Queue__JKI_lib_State_Machine.vi"("State(s) in Front (\"\")"="Loading Macro: Initialize" ("State(s) in Front (\"\")"), "State(s) in (\"\")"=w876) -> ("States Out"=w875:string)  [unwired: 13 in]
      }
      frame "Loading Macro: Initialize" {
        # "Do not put any code in this frame.\n(It is a separator no-op. You can make a copy of this frame to create a new UI frame)"
        n334 = call <vilib>:"Add State(s) to Queue__JKI_lib_State_Machine.vi"("State(s) in (\"\")"=w880) -> ("States Out"=w879:string)  [unwired: 14 in]
      }
      frame "---------- cDAQ ----------" {
        # "Do not put any code in this frame.\n(It is a separator no-op. You can make a copy of this frame to create a new Data frame)"
        n335 = call <vilib>:"Add State(s) to Queue__JKI_lib_State_Machine.vi"("State(s) in (\"\")"=w884) -> ("States Out"=w883:string)  [unwired: 14 in]
      }
      frame "cDAQ: Scan" {
        # "Scan for cDAQ IDs\n(this is called automatically, by the Connections: Initialize)"
        n336 = call "CDAQ_Scan.vi"("DataCluster"=w886) -> ("DataCluster out"=w885:T1)  [unwired: 10 in]
        n337 = call <vilib>:"Add State(s) to Queue__JKI_lib_State_Machine.vi"("State(s) in (\"\")"=w889) -> ("States Out"=w888:string)  [unwired: 14 in]
      }
      frame "cDAQ: Initialize" {
        # "Initialize the System Connections, here.\n(this is called automatically, by the Macro: Init)"
        n338 = call "Pt100_Config.vi"("error in (no error)"=w890, "DataCluster in"=w893) -> ("error out"=w891:errorcluster, "State out"=w892:string, "DataCluster out"=w894:T1)  [unwired: 7 in]
        n339 = call <vilib>:"Add State(s) to Queue__JKI_lib_State_Machine.vi"("State(s) in Front (\"\")"=w892, "State(s) in (\"\")"=w896) -> ("States Out"=w895:string)  [unwired: 13 in]
      }
      frame "cDAQ: Terminate" {
        # "Terminate connection to DAQs and Power Supply (Peltier)"
        # "Terminate the System Connections, here.\n(this is called automatically, by the Macro: Exit)"
        n340 = Unbundle By Name(w900) -> ("Connections.cDAQ.Task"=w901:refnum<k21>, "Connections.cDAQ.Connected"=w902:bool)
        n341 = case shown="True" w902 {
          tunnel: w901 -> [_ w909]
          tunnel: w900 -> [w906 w912]
          tunnel: [w906 w911] -> w899
          tunnel: [w905 w910] -> w898
          tunnel: w897 -> [w905 w908]
          frame False {
          }
          frame True {
            w907 = FALSE ("Connections.cDAQ.Connected")
            n342 = call <vilib>:"DAQmx Clear Task.vi"("task in"=w909, "error in"=w908) -> ("error out"=w910:errorcluster)  [unwired: 13 in]
            n343 = Bundle By Name(cluster=w912, "Connections.cDAQ.Connected"=w907, "Connections.cDAQ.Active"=w907) -> (w911:T1)
          }
        }
        n344 = call <vilib>:"Add State(s) to Queue__JKI_lib_State_Machine.vi"("State(s) in (\"\")"=w904) -> ("States Out"=w903:string)  [unwired: 14 in]
      }
      frame "---------- Camera ----------" {
        # "Do not put any code in this frame.\n(It is a separator no-op. You can make a copy of this frame to create a new Data frame)"
        n345 = call <vilib>:"Add State(s) to Queue__JKI_lib_State_Machine.vi"("State(s) in (\"\")"=w916) -> ("States Out"=w915:string)  [unwired: 14 in]
      }
      frame "Camera: Initialize" {
        # "Setup connection to Cam"
        # "Initialize the System Connections, here.\n(this is called automatically, by the Macro: Init)"
        n346 = call "TCam_Scan.vi"("input cluster"=w920) -> ("error out"=w917:errorcluster, "State out"=w918:string, "output cluster"=w919:T1)  [unwired: 8 in]
        n347 = call <vilib>:"Add State(s) to Queue__JKI_lib_State_Machine.vi"("State(s) in Front (\"\")"=w918, "State(s) in (\"\")"=w922) -> ("States Out"=w921:string)  [unwired: 13 in]
      }
      frame "Camera: Terminate" {
        # "Terminate connection to Thermal Camear"
        # "Terminate the System Connections, here.\n(this is called automatically, by the Macro: Exit)"
        n348 = Unbundle By Name(w926) -> ("Connections.Camera.Session"=w927:T2, "Connections.Camera.Connected"=w928:bool)
        n349 = case shown="True" w928 {
          tunnel: w927 -> [_ w935]
          tunnel: w926 -> [w932 w938]
          tunnel: [w932 w936] -> w925
          tunnel: [w931 w934] -> w924
          tunnel: w923 -> [w931 w933]
          frame False {
          }
          frame True {
            n350 = call <vilib>:"IMAQdx Close Camera.vi"("error in"=w933, "Session In"=w935) -> ("error out"=w934:errorcluster)  [unwired: 9 in]
            n351 = Bundle By Name(cluster=w938, "Connections.Camera.Connected"=FALSE ("Connections.cDAQ.Connected")) -> (w936:T1)
          }
        }
        n352 = call <vilib>:"Add State(s) to Queue__JKI_lib_State_Machine.vi"("State(s) in (\"\")"=w930) -> ("States Out"=w929:string)  [unwired: 14 in]
      }
      frame "---------- Arduino ----------" {
        # "Do not put any code in this frame.\n(It is a separator no-op. You can make a copy of this frame to create a new Data frame)"
        n353 = call <vilib>:"Add State(s) to Queue__JKI_lib_State_Machine.vi"("State(s) in (\"\")"=w942) -> ("States Out"=w941:string)  [unwired: 14 in]
      }
      frame "Arduino: Initialize" {
        # "Initialize Arduino Connections, here.\n(this is called automatically, by the Connections: Initialize)"
        n354 = call "Arduino_Initialize.vi"("DataCluster"=w946) -> ("error out"=w943:errorcluster, "State out"=w944:string, "output cluster"=w945:T1)  [unwired: 8 in]
        n355 = call <vilib>:"Add State(s) to Queue__JKI_lib_State_Machine.vi"("State(s) in Front (\"\")"=w944, "State(s) in (\"\")"=w948) -> ("States Out"=w947:string)  [unwired: 13 in]
      }
      frame "Arduino: Mode" {
        # "Initialize Arduino Connections, here.\n(this is called automatically, by the Connections: Initialize)"
        n356 = call "Arduino_Mode.vi"("Arguments"=w951, "input cluster"=w953) -> ("error out"=w949:errorcluster, "State out"=w950:string, "Output Clustesr"=w952:T1)  [unwired: 7 in]
        n357 = call <vilib>:"Add State(s) to Queue__JKI_lib_State_Machine.vi"("State(s) in Front (\"\")"=w950, "State(s) in (\"\")"=w955) -> ("States Out"=w954:string)  [unwired: 13 in]
      }
      frame "Arduino: Terminate" {
        # "Initialize Arduino Connections, here.\n(this is called automatically, by the Connections: Initialize)"
        n358 = Unbundle By Name(w959) -> ("Connections.Arduino.Port"=w960:refnum<visa-resource-name>, "Connections.Arduino.Connected"=w961:bool)
        n359 = case shown="True" w961 {
          tunnel: w960 -> [_ w971]
          tunnel: w959 -> [w965 w970]
          tunnel: [w965 w968] -> w958
          tunnel: [w964 w967] -> w957
          tunnel: w956 -> [w964 w966]
          frame False {
          }
          frame True {
            w969 = FALSE ("Connections.Arduino.Connected")
            n360 = VISA Close(VISA resource name=w971, error in (no error)=w966) -> (error out=w967:errorcluster)
            n361 = Bundle By Name(cluster=w970, "Connections.Arduino.Connected"=w969, "Connections.Arduino.Active"=w969) -> (w968:T1)
          }
        }
        n362 = call <vilib>:"Add State(s) to Queue__JKI_lib_State_Machine.vi"("State(s) in (\"\")"=w963) -> ("States Out"=w962:string)  [unwired: 14 in]
      }
      frame "---------- PSU ----------" {
        # "Template Separator\n(You can make a copy of, or modify, this frame)"
        n363 = call <vilib>:"Add State(s) to Queue__JKI_lib_State_Machine.vi"("State(s) in (\"\")"=w975) -> ("States Out"=w974:string)  [unwired: 14 in]
      }
      frame "PSU: Mode" {
        # "Template Separator\n(You can make a copy of, or modify, this frame)"
        n364 = Unbundle By Name(w978) -> ("Connections.PSU.Connected"=w977:bool)
        n365 = case shown="True" w977 {
          tunnel: w978 -> [w986 w991]
          tunnel: w982 -> [_ w990]
          tunnel: [w985 w987] -> w981
          tunnel: [_ w988] -> w980
          tunnel: [w986 w989] -> w979
          tunnel: w976 -> [w985 w987]
          frame False {
          }
          frame True {
            n366 = call "PSU_State.vi"("Arguments"=w990, "DataCluster"=w991) -> ("State(s) in Front (\"\")"=w988:string, "DataCluster out"=w989:T1)  [unwired: 7 in, 1 out]
          }
        }
        n367 = call <vilib>:"Add State(s) to Queue__JKI_lib_State_Machine.vi"("State(s) in Front (\"\")"=w980, "State(s) in (\"\")"=w984) -> ("States Out"=w983:string)  [unwired: 13 in]
      }
      frame "PSU: Output" {
        # "Template Separator\n(You can make a copy of, or modify, this frame)"
        n368 = case shown="\"OFF\", Default" w993 {
          tunnel: [0 70] -> w994
          frame "OFF", Default {
          }
          frame "ON" {
          }
        }
        n369 = Unbundle By Name(w995) -> ("Connections.PSU.Connected"=w997:bool)
        n370 = case shown="True" w997 {
          tunnel: w995 -> [_ w1009]
          tunnel: w994 -> [_ w1008]
          tunnel: [w1003 w1007] -> w998
          tunnel: [_ w1006] -> w996
          tunnel: w992 -> [w1003 w1004]
          frame False {
          }
          frame True {
            n371 = call "PSU_Output.vi"("error in (no error)"=w1004, "CheckResponse?"=TRUE, "Output %"=w1008, "DataCluster in"=w1009) -> ("error out"=w1007:errorcluster, "Output % duplicate"=w1006:dbl)  [unwired: 5 in, 1 out]
          }
        }
        n372 = local write "Cooling%"(w996) -> ()
        n373 = call <vilib>:"Add State(s) to Queue__JKI_lib_State_Machine.vi"("State(s) in (\"\")"=w1000) -> ("States Out"=w999:string)  [unwired: 14 in]
      }
      frame "PSU: Initialize" {
        # "Setup connection to PSU"
        # "Initialize the System Connections, here.\n(this is called automatically, by the Macro: Init)"
        n374 = call "VISA_Scan.vi"("error in (no error)"=w1010, "DataCluster"=w1013) -> ("error out"=w1011:errorcluster, "State out"=w1012:string, "DataCluster out"=w1014:T1)  [unwired: 6 in, 1 out]
        n375 = call <vilib>:"Add State(s) to Queue__JKI_lib_State_Machine.vi"("State(s) in Front (\"\")"=w1012, "State(s) in (\"\")"=w1016) -> ("States Out"=w1015:string)  [unwired: 13 in]
      }
      frame "PSU: Terminate" {
        # "Terminate the System Connections, here.\n(this is called automatically, by the Macro: Exit)"
        n376 = Unbundle By Name(w1020) -> ("Connections.PSU.Port"=w1021:refnum<visa-resource-name>, "Connections.PSU.Connected"=w1022:bool)
        n377 = case shown="True" w1022 {
          tunnel: w1021 -> [_ w1029]
          tunnel: w1020 -> [w1026 w1032]
          tunnel: [w1026 w1030] -> w1019
          tunnel: [w1025 w1028] -> w1018
          tunnel: w1017 -> [w1025 w1027]
          frame False {
          }
          frame True {
            n378 = VISA Close(VISA resource name=w1029, error in (no error)=w1027) -> (error out=w1028:errorcluster)
            n379 = Bundle By Name(cluster=w1032, "Connections.PSU.Connected"=FALSE ("Connections.cDAQ.Connected")) -> (w1030:T1)
          }
        }
        n380 = call <vilib>:"Add State(s) to Queue__JKI_lib_State_Machine.vi"("State(s) in (\"\")"=w1024) -> ("States Out"=w1023:string)  [unwired: 14 in]
      }
      frame "---------- Data Acquisition ----------" {
        # "Template Separator\n(You can make a copy of, or modify, this frame)"
        n381 = call <vilib>:"Add State(s) to Queue__JKI_lib_State_Machine.vi"("State(s) in (\"\")"=w1036) -> ("States Out"=w1035:string)  [unwired: 14 in]
      }
      frame "Data Acquisition: Start" {
        # "Access Data Setup here.\n(this is called automatically, by the Settings Event Run time menu)"
        n382 = Unbundle By Name(w1037) -> ("Data Acquisition.Ready"=w1043:bool, "Data Acquisition.Active"=w1042:bool)
        n383 = Not(x=w1042) -> (.not. x?=w1044:bool)
        n384 = And(x=w1043, y=w1044) -> (x .and. y?=w1038:bool)
        n385 = case shown="False" w1038 {
          selector: w1038 -> [w1050 _]
          tunnel: [w1049 _] -> w1040
          tunnel: w1037 -> [w1048 w1055]
          tunnel: [w1048 w1053] -> w1041
          tunnel: w1043 -> [w1047 _]
          frame False {
            n386 = local write "Start"(w1050) -> ()
            n387 = case shown="False" w1047 {
              tunnel: ["UI: Connections Status" ("State(s) in Front (\"\")") "" ("State(s) in Front (\"\")")] -> w1049
              frame False {
              }
              frame True {
              }
            }
          }
          frame True {
            n388 = Bundle By Name(cluster=w1055, "Data Acquisition.Active"=TRUE ("System.Active")) -> (w1053:T1)
          }
        }
        n389 = call <vilib>:"Add State(s) to Queue__JKI_lib_State_Machine.vi"("State(s) in Front (\"\")"=w1040, "State(s) in (\"\")"=w1046) -> ("States Out"=w1045:string)  [unwired: 13 in]
      }
      frame "Data Acquisition: cDAQ Initialize" {
        # "Your code here.\n(You can make a copy of, or modify, this frame)"
        n390 = Unbundle By Name(w1062) -> ("Connections.cDAQ.Task"=w1064:refnum<k21>, "Connections.cDAQ.Connected"=w1060:bool, "Connections.cDAQ.Active"=w1058:bool)
        n391 = Not(x=w1058) -> (.not. x?=w1057:bool)
        n392 = And(x=w1060, y=w1057) -> (x .and. y?=w1059:bool)
        n393 = case shown="True" w1059 {
          tunnel: w1064 -> [_ w1075]
          tunnel: [w1067 w1071] -> w1063
          tunnel: w1062 -> [w1068 w1073]
          tunnel: [w1068 w1072] -> w1061
          tunnel: w1056 -> [w1067 w1070]
          frame False {
          }
          frame True {
            n394 = call <vilib>:"DAQmx Start Task.vi"("task/channels in"=w1075, "error in"=w1070) -> ("task out"=w1069:refnum<k21>, "error out"=w1071:errorcluster)  [unwired: 12 in]
            n395 = Bundle By Name(cluster=w1073, "Connections.cDAQ.Active"=TRUE ("Connections.Camera.Active"), "Connections.cDAQ.Task"=w1069) -> (w1072:T1)
          }
        }
        n396 = call <vilib>:"Add State(s) to Queue__JKI_lib_State_Machine.vi"("State(s) in (\"\")"=w1066) -> ("States Out"=w1065:string)  [unwired: 14 in]
      }
      frame "Data Acquisition: cDAQ Terminate" {
        # "Your code here.\n(You can make a copy of, or modify, this frame)"
        n397 = Unbundle By Name(w1079) -> ("Connections.cDAQ.Connected"=w1076:bool, "Connections.cDAQ.Task"=w1081:refnum<k21>)
        n398 = case shown="True" w1076 {
          tunnel: w1081 -> [_ w1091]
          tunnel: [w1084 w1090] -> w1080
          tunnel: w1079 -> [w1085 w1088]
          tunnel: [w1085 w1087] -> w1078
          tunnel: w1077 -> [w1084 w1086]
          frame False {
          }
          frame True {
            n399 = call <vilib>:"DAQmx Stop Task.vi"("task/channels in"=w1091, "error in"=w1086) -> ("error out"=w1090:errorcluster)  [unwired: 12 in, 1 out]
            n400 = Bundle By Name(cluster=w1088, "Connections.cDAQ.Active"=FALSE ("Connections.Camera.Active")) -> (w1087:T1)
          }
        }
        n401 = call <vilib>:"Add State(s) to Queue__JKI_lib_State_Machine.vi"("State(s) in (\"\")"=w1083) -> ("States Out"=w1082:string)  [unwired: 14 in]
      }
      frame "Data Acquisition: Camera Initialize" {
        # "Your code here.\n(You can make a copy of, or modify, this frame)"
        n402 = Unbundle By Name(w1094) -> ("Connections.Camera.Connected"=w1093:bool)
        n403 = case shown="True" w1093 {
          tunnel: [w1100 w1104] -> w1096
          tunnel: [w1099 w1103] -> w1095
          tunnel: w1094 -> [w1100 w1105]
          tunnel: w1092 -> [w1099 w1101]
          frame False {
          }
          frame True {
            n404 = call "TCam_Config.vi"("error in (no error)"=w1101, "crop?"=TRUE, "DataCluster in"=w1105) -> ("error out"=w1103:errorcluster, "DataCluster out"=w1104:T1)  [unwired: 7 in]
          }
        }
        n405 = call <vilib>:"Add State(s) to Queue__JKI_lib_State_Machine.vi"("State(s) in (\"\")"=w1098) -> ("States Out"=w1097:string)  [unwired: 14 in]
      }
      frame "Data Acquisition: Camera Terminate" {
        # "Your code here.\n(You can make a copy of, or modify, this frame)"
        n406 = Unbundle By Name(w1110) -> ("Data Acquisition.Camera.Image"=w1107:T3, "Connections.Camera.Session"=w1112:T2, "Connections.Camera.Connected"=w1108:bool)
        n407 = case shown="True" w1108 {
          tunnel: w1112 -> [_ w1126]
          tunnel: w1111 -> [w1115 w1125]
          tunnel: w1110 -> [w1116 w1124]
          tunnel: [w1116 w1122] -> w1109
          tunnel: w1107 -> [_ w1119]
          tunnel: [w1115 w1117] -> w1106
          frame False {
          }
          frame True {
            n408 = call <vilib>:"IMAQdx Unconfigure Acquisition.vi"("error in"=w1125, "Session In"=w1126) -> ("error out"=w1121:errorcluster, "Session Out"=w1120:T2)  [unwired: 8 in]
            n409 = call <vilib>:"IMAQdx Stop Acquisition.vi"("error in"=w1121, "Session In"=w1120) -> ("error out"=w1118:errorcluster)  [unwired: 8 in, 1 out]
            n410 = Bundle By Name(cluster=w1124, "Connections.Camera.Active"=FALSE) -> (w1122:T1)
            n411 = call "IMAQ Dispose"("Image"=w1119, "error in (no error)"=w1118) -> ("error out"=w1117:errorcluster)  [unwired: 4 in]
          }
        }
        n412 = call <vilib>:"Add State(s) to Queue__JKI_lib_State_Machine.vi"("State(s) in (\"\")"=w1114) -> ("States Out"=w1113:string)  [unwired: 14 in]
      }
      frame "Data Acquisition: Buffer Initialize" {
        # "Access Data Setup here.\n(this is called automatically, by the Settings Event Run time menu)"
        n413 = call "Buffer_Initialize.vi"("error in (no error)"=w1129, "DataCluster in"=w1130) -> ("error out"=w1128:errorcluster, "DataCluster Out"=w1127:T1)  [unwired: 8 in]
        n414 = call <vilib>:"Add State(s) to Queue__JKI_lib_State_Machine.vi"("State(s) in (\"\")"=w1132) -> ("States Out"=w1131:string)  [unwired: 14 in]
      }
      frame "Data Acquisition: Buffer Terminate" {
        # "Access Data Setup here.\n(this is called automatically, by the Settings Event Run time menu)"
        n415 = Unbundle By Name(w1133) -> ("Data Acquisition.Queue.Queue"=w1134:refnum<queue>)
        n416 = Release Queue(queue=w1134, force destroy? (F)=FALSE, error in (no error)=w1136) -> (error out=w1135:errorcluster)  [unwired: 2 out]
        n417 = call <vilib>:"Add State(s) to Queue__JKI_lib_State_Machine.vi"("State(s) in (\"\")"=w1139) -> ("States Out"=w1138:string)  [unwired: 14 in]
      }
      frame "---------- Tools ----------" {
        # "Template Separator\n(You can make a copy of, or modify, this frame)"
        n418 = call <vilib>:"Add State(s) to Queue__JKI_lib_State_Machine.vi"("State(s) in (\"\")"=w1143) -> ("States Out"=w1142:string)  [unwired: 14 in]
      }
      frame "Tools: Sensor Readout" {
        # "Your code here.\n(You can make a copy of, or modify, this frame)"
        n419 = call "Thermistor_Manual_Read.vi"("error in"=w1146, "temp readings"=w1144, "input cluster"=w1147) -> ("error out"=w1145:errorcluster)  [unwired: 7 in, 1 out]
        n420 = call <vilib>:"Add State(s) to Queue__JKI_lib_State_Machine.vi"("State(s) in (\"\")"=w1149) -> ("States Out"=w1148:string)  [unwired: 14 in]
      }
      frame "Tools: Camera Feed" {
        # "Your code here.\n(You can make a copy of, or modify, this frame)"
        n421 = call "Camera_Feed.vi"("error in"=w1153, "DataCluster"=w1154) -> ("error out"=w1152:errorcluster, "DataCluster out"=w1151:T1)  [unwired: 8 in]
        n422 = call <vilib>:"Add State(s) to Queue__JKI_lib_State_Machine.vi"("State(s) in Front (\"\")"="UI: StatusString >> Initializing Camera\nData Acquisition: Camera Initialize\nUI: Cursor Set >> Idle\nUI: StatusString >> Idle" ("State(s) in Front (\"\")"), "State(s) in (\"\")"=w1156) -> ("States Out"=w1155:string)  [unwired: 13 in]
      }
      frame "Tools: Focus Thermal Camera" {
        # "Your code here.\n(You can make a copy of, or modify, this frame)"
        n423 = call "TCam_AutoFocus.vi"("error in (no error)"=w1160, "DataCluster in"=w1158) -> ("error out"=w1159:errorcluster, "DataCluster out"=w1157:T1)  [unwired: 8 in]
        n424 = call <vilib>:"Add State(s) to Queue__JKI_lib_State_Machine.vi"("State(s) in (\"\")"=w1162) -> ("States Out"=w1161:string)  [unwired: 14 in]
      }
      frame "Tools: PID" {
        # "Your code here.\n(You can make a copy of, or modify, this frame)"
        n425 = call "Manual_Cool_Heat.vi"("error in"=w1166, "input cluster"=w1167) -> ("error out"=w1165:errorcluster, "State out"=w1163:string, "input cluster out"=w1164:T1)  [unwired: 7 in]
        n426 = call <vilib>:"Add State(s) to Queue__JKI_lib_State_Machine.vi"("State(s) in Front (\"\")"=w1163, "State(s) in (\"\")"=w1169) -> ("States Out"=w1168:string)  [unwired: 13 in]
      }
      frame "Tools: Manual Temp Control" {
        # "Your code here.\n(You can make a copy of, or modify, this frame)"
        n427 = call "Manual_Cool_Heat_V2.vi"("error in"=w1172, "DataCluster"=w1170) -> ("error out"=w1171:errorcluster)  [unwired: 9 in]
        n428 = call <vilib>:"Add State(s) to Queue__JKI_lib_State_Machine.vi"("State(s) in (\"\")"=w1174) -> ("States Out"=w1173:string)  [unwired: 14 in]
      }
      frame "Tools: Freeze Check" {
        # "Access Data Setup here.\n(this is called automatically, by the Settings Event Run time menu)"
        n429 = call "Freeze_Check.vi"("error in (no error)"=w1176, "DataCluster in"=w1177) -> ("error out"=w1175:errorcluster)  [unwired: 9 in]
        n430 = call <vilib>:"Add State(s) to Queue__JKI_lib_State_Machine.vi"("State(s) in (\"\")"=w1179) -> ("States Out"=w1178:string)  [unwired: 14 in]
      }
      frame "Tools: Calibrate Thermal Camera" {
        # "Your code here.\n(You can make a copy of, or modify, this frame)"
        n431 = call <vilib>:"Application Directory.vi"() -> ("Application Directory"=w1184:path)
        n432 = Build Path(base path=w1184, name or relative path=path "TCC.exe") -> (appended path=w1182:path)
        n433 = Path To String(path=w1182) -> (string=w1181:string)
        n434 = call <vilib>:"System Exec.vi"("run minimized? (F)"=TRUE, "wait until completion? (T)"=FALSE, "command line"=w1181) -> ()  [unwired: 5 in, 4 out]
        n435 = call <vilib>:"Add State(s) to Queue__JKI_lib_State_Machine.vi"("State(s) in (\"\")"=w1189) -> ("States Out"=w1188:string)  [unwired: 14 in]
      }
      frame "Tools: Temp Calc" {
        # "Access Data Setup here.\n(this is called automatically, by the Settings Event Run time menu)"
        n436 = call <vilib>:"Application Directory.vi"() -> ("Application Directory"=w1190:path)
        n437 = Build Path(base path=w1190, name or relative path=path "TCE.exe") -> (appended path=w1195:path)
        n438 = Path To String(path=w1195) -> (string=w1194:string)
        n439 = call <vilib>:"System Exec.vi"("run minimized? (F)"=TRUE, "wait until completion? (T)"=FALSE, "command line"=w1194) -> ("error out"=→"error out 2":errorcluster)  [unwired: 5 in, 3 out]
        n440 = call <vilib>:"Add State(s) to Queue__JKI_lib_State_Machine.vi"("State(s) in (\"\")"=w1200) -> ("States Out"=w1199:string)  [unwired: 14 in]
      }
    }
    n441 = call "LoadingWindow_Stream.vi"("DataCluster"=w9, "Arguments"=w10, "Current State"=w24) -> ("Channel out"=w11:T14)
    n442 = call "DAQ_Status_Read.vi"("channel"=w13) -> ("state"=w8:string)
    n443 = call <vilib>:"Add State(s) to Queue__JKI_lib_State_Machine.vi"("State(s) in (\"\")"=w16, "State(s) at Back (\"\")"=w8) -> ("States Out"=w15:string)  [unwired: 13 in]
    n444 = call <extravilib>:"Write.vi"("element"=w12) -> ("channel"=w17:T15)  [unwired: 1 out]
  }
  n445 = call "LoadingWindow.vi"("channel"=w2) -> ()  [unwired: 11 in]
  n446 = while "Data Logging Loop" {
    tunnel: w1 -> [w1206]
    tunnel: w1 -> [w1205]
    stop <- w1204 stop-if-true
    n447 = call <extravilib>:"Read.vi"("channel"=w1206) -> ("element"=w1203:T1)  [unwired: 1 in, 1 out]
    n448 = call "Camera_Frequency.vi"("DataCluster"=w1203) -> ("Image Frequency"=w1202:i32)
    n449 = call "SystemActive.vi"("DataCluster"=w1203) -> ("Exit"=w1204:bool, "Active"=w1201:bool)  [unwired: 1 in, 5 out]
    n450 = case shown="True" w1201 {
      tunnel: w1205 -> [_ w1212]
      tunnel: w1202 -> [_ w1211]
      frame False {
        # "Data Acquisition Idle"
        n451 = Wait (ms)(milliseconds to wait=u32 100) -> ()  [unwired: 1 out]
      }
      frame True {
        # "Data Acquisition Active"
        n452 = node-c288(i64 50 ("Period")) -> (w1210:T16)  [unwired: 1 in]
        n453 = timed-loop {
          tunnel: w1212 -> [w1218]
          shift-right: [w1214] -> _
          shift-left: w1211 -> [w1215]
          timing: w1210 -> [_]
          timing-out: [_] -> w1209
          stop <- w1217 stop-if-true
          # "Active Data Logging Loop"
          n454 = node-c288() -> ()  [unwired: 1 in]
          n455 = call <extravilib>:"Read.vi"("channel"=w1218) -> ("element"=w1213:T1)  [unwired: 1 in, 1 out]
          n456 = call "SystemActive.vi"("DataCluster"=w1213) -> ("!Ready/!Active/Exit"=w1217:bool)  [unwired: 1 in, 6 out]
          n457 = call "DataFile_Append.vi"("iteration"=w1215, "DataCluster"=w1213) -> ("iteration out"=w1214:i32)  [unwired: 9 in]
          n458 = node-c288() -> ()  [unwired: 1 out]
          n459 = Wait (ms)(milliseconds to wait=u32 50) -> ()  [unwired: 1 out]
        }
        n460 = node-c288(w1209) -> ()  [unwired: 1 out]
      }
    }
  }
  n461 = while "Data Acquisition Loop" {
    tunnel: w1 -> [w1231]
    tunnel: w1 -> [w1230]
    tunnel: [w1227] -> w4
    tunnel: [w1226] -> w3
    stop <- w1229 stop-if-true
    n462 = call <extravilib>:"Read.vi"("channel"=w1231) -> ("element"=w1228:T1)  [unwired: 1 in, 1 out]
    n463 = call "SystemActive.vi"("DataCluster"=w1228) -> ("Exit"=w1229:bool, "Ready"=w1225:bool)  [unwired: 1 in, 5 out]
    n464 = case shown="True" w1225 {
      tunnel: w1230 -> [_ w1240]
      tunnel: w1228 -> [_ w1237]
      tunnel: [_ w1233] -> w1227
      tunnel: [_ w1235] -> w1226
      frame False {
        # "System not Ready"
        n465 = Wait (ms)(milliseconds to wait=u32 100) -> ()  [unwired: 1 out]
      }
      frame True {
        # "System Ready"
        n466 = call "SampleRate_Convert.vi"("DataCluster"=w1237) -> ("Sample dt (ms)"=w1234:i64)  [unwired: 1 out]
        n467 = node-c288(w1234) -> (w1239:T16)  [unwired: 1 in]
        n468 = timed-loop {
          tunnel: w1240 -> [w1256]
          timing: w1239 -> [_]
          timing-out: [_] -> w1238
          shift-right: [w1251] -> _
          shift-left: cluster{dbl[], dbl[], dbl[], dbl[], dbl[][]} {[], [], [], [], []} ("Data Cluster in") -> [w1249]
          tunnel: [w1255] -> w1235
          tunnel: w1234 -> [_]
          tunnel: [w1248] -> w1233
          stop <- w1242 stop-if-true
          n469 = node-c288() -> (w1250:i64)  [unwired: 1 in]
          n470 = call "DAQ_Control.vi"("Channel in"=w1256, "Reading Cluster in"=w1249, "Iteration Duration"=w1250) -> ("DAQ time"=→"cDAQ_Time":u32, "Gradients"=→"Gradients":waveform(dbl)[], "cDAQ time"=→"DL_Time":u32, "Stop?"=w1242:bool, "Temps"=→"Temps":waveform(dbl)[], "Time Left:"=→"T_Left":string, "Camera Feed"=→"Camera Feed":T3, "Output%"=→"Cooling%":dbl, "Channel out"=w1255:T14, "Readings out"=w1248:T19, "Reading Cluster"=w1251:T20, "DP_Overhead"=→"DP_Overhead":i64, "Temp"=→"Temp":dbl[unit])  [unwired: 4 in]
          n471 = node-c288() -> ()  [unwired: 1 out]
        }
        n472 = node-c288(w1238) -> ()
      }
    }
  }
